vi "Parser Dryer Performance.vi"(8 "error in":errorcluster, 9 "Process Debug?":bool, 10 "log file path in":path=path "C:/faildryer/T00063280_12HL1942_12lb_   COT_R150_ 90IMC_2 - _dlr_run   5_75 50_20120702_1508_DPT.csv", 11 "debug log path in":path=path "C:/test1/dubuglogtest.csv") -> (0 "error out":errorcluster, 2 "new file path out":path)   [LabVIEW 2012]
uses:
  Global Test Variables DPT.vi
  <vilib>/Analysis/baseanly.llb/Mean (DBL).vi
  <vilib>/Utility/file.llb/Write To Spreadsheet File (string).vi
  <vilib>/gmath/NI_Gmath.lvlib
  <vilib>/Analysis/NI_AALBase.lvlib
panel:
  in  "analysis file":path=path "C:/Documents and Settings/JOHN CONWAY/Desktop/Cham 2 Failures/Analysis.csv"
  in  "Write Analysis File":bool
  out "File Name String":string
  out "Compensated - raw":cluster{"Column Data":dbl[], dbl[]}(graph)
  in  "Debug Information":enum32{"Debug Info", "Page 2"}(tab)
  out "Timeing":u32[](array[numeric])
  out "Array":string[](array[string])
  out "Current State":string
  out "Date Time String Array":string[][](array[string])
  out "Debug Time Array":string[](array[string])
  in  "Write Eng File?":bool=TRUE
  in  "Tab Control":T1(tab)=enum."Debug Log"
  out "Data Log File Data In":string[][](array[string])
  out "File Data Out":string[][](array[string])
  in  "Filename Suffix":string="_ENG"
  out "TT4 Extrapolated":bool
  out "RMC Compensated":T2(graph)
  out "Init Moisture Content":dbl
  out "Final Moisture %":dbl
  out "Date String":string
  out "RDB F":T3(graph)
  out "TT 3%":dbl
  out "TT 4%":dbl
  out "TT 5%":dbl
  out "TT3 Extrapolated":bool
  out "TT5 Extrapolated":bool
  out "Gas kWH":T3(graph)
  out "Total kWH":T3(graph)
  out "Heating Val":dbl
  out "Electric kWH":T3(graph)
  out "Total kWH":dbl
  out "Elec kWH":dbl
  out "Gas kWH 2":dbl
  out "Electric Watts":T3(graph)
  out "Gas Watts":T3(graph)
  out "Ave Gas Watts":dbl format="%0.2f"
  out "Ave Elect Watts":dbl format="%0.2f"
  out "Com Count (x(k+1)-x(k))":dbl[](graph)
  out "Debug Data":dbl[][](array[numeric])
  out "Headers for Debug Data":string[](array[string])
  out "error out":errorcluster
  out "Error Indicated in Last 2cols\nof Debug Log":bool
  out "Weight/Raw Weight Data":T2(graph)
  out "FMC (lbs)":dbl
  out "Empty Dryer Wt":dbl
  out "Measured IMC":dbl
  out "FMC %":dbl
  out "FMC (lbs) Predicted":dbl
  out "BDW":dbl
  out "Gas W Data":dynamicdata(graph)
  out "Gas Temp E38":dbl[](array[numeric])
  out "Gas Vol Init E41":dbl
  out "Gas Vol E42":dbl[](array[numeric])
  out "Gas Pres E37":dbl[](array[numeric])
  out "Bar.Pres E36":dbl[](array[numeric])
  out "Header":string[](array[string])
  in  "OK":bool
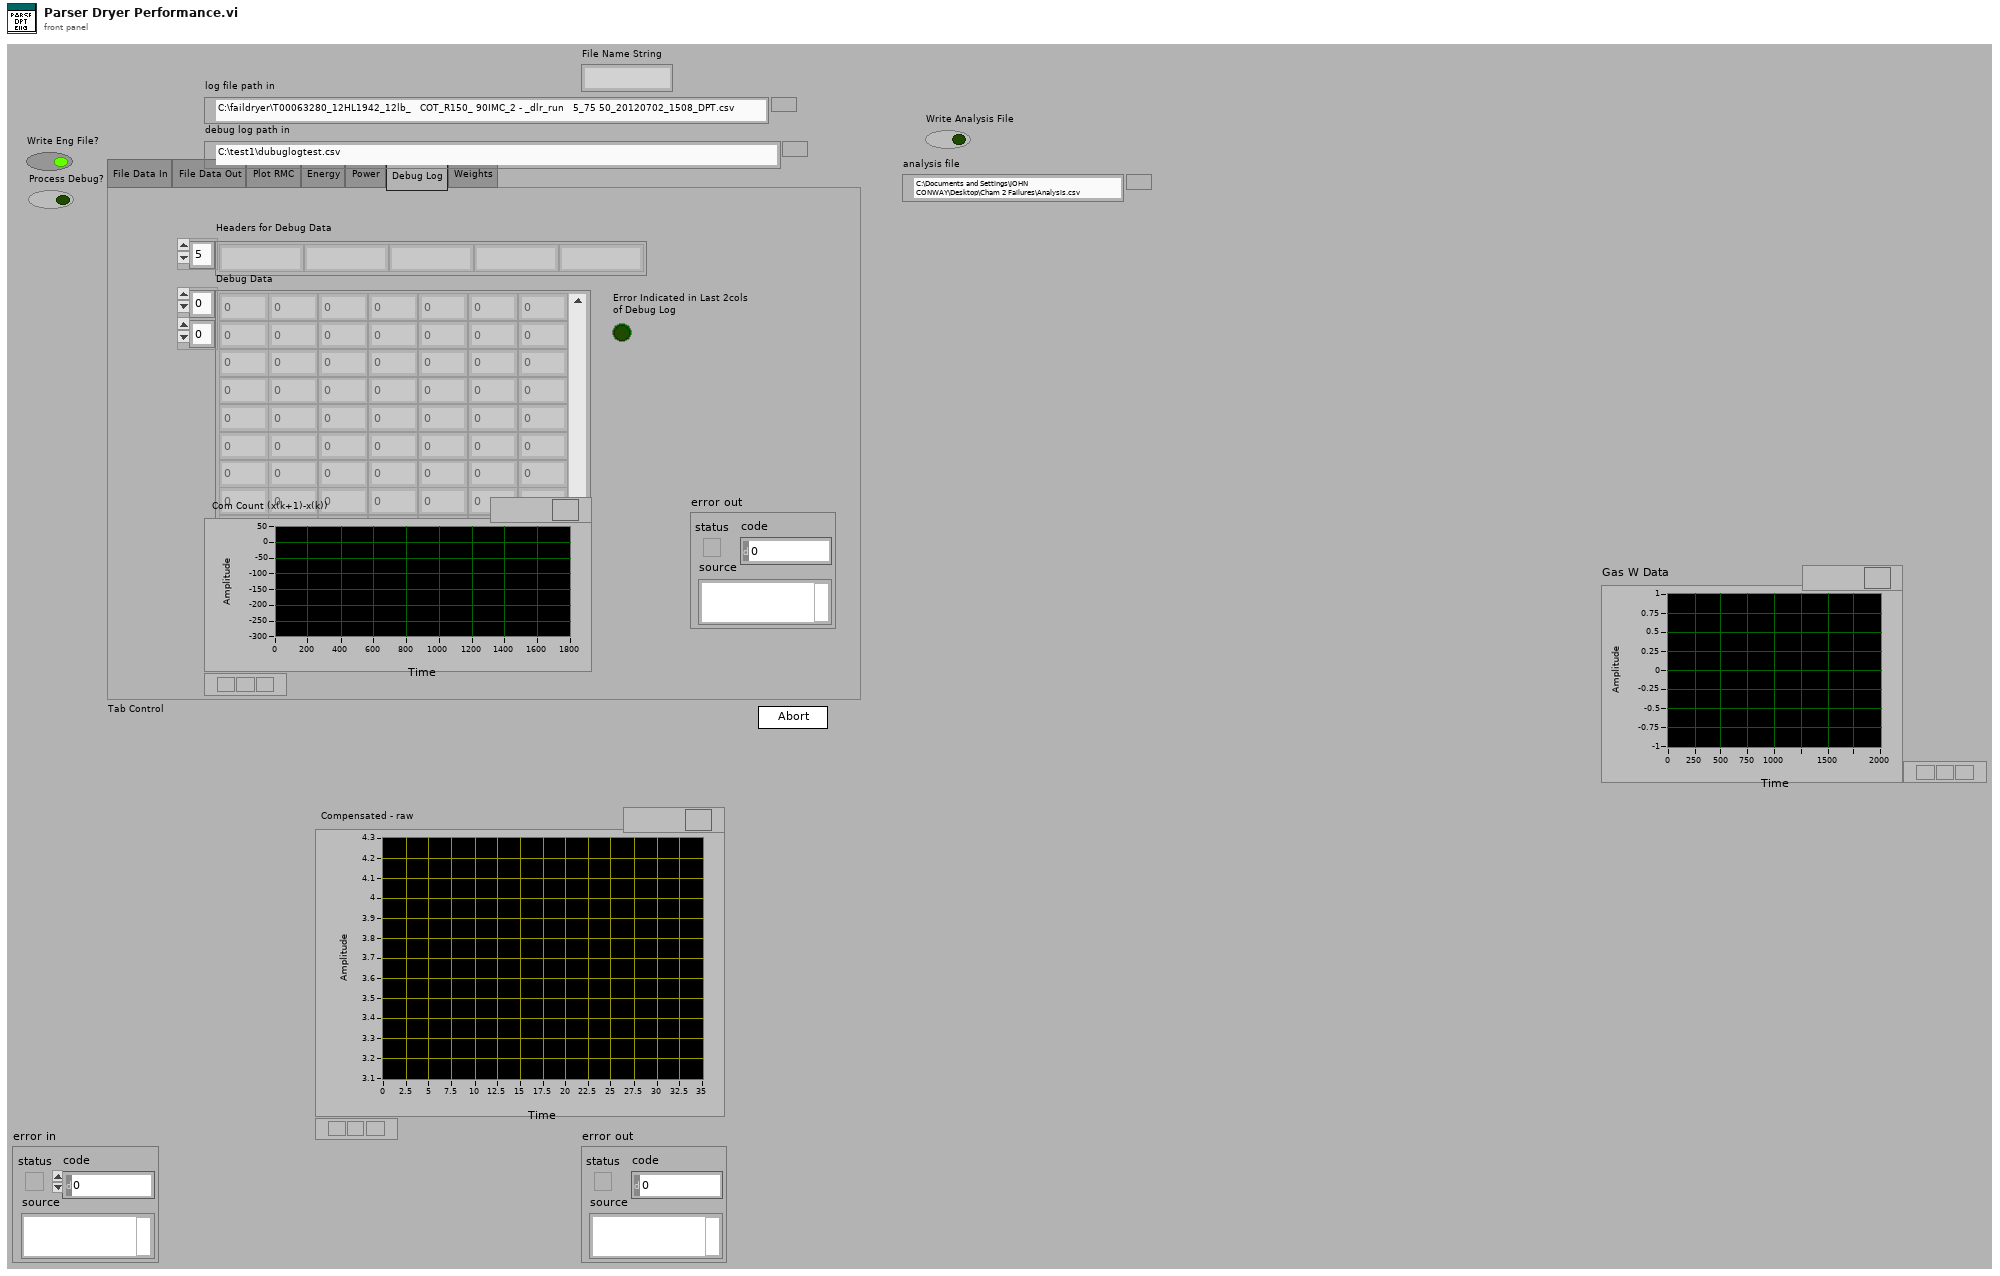
[diagram p1: front panel]
types:
  T1 = enum32{"File Data In", "File Data Out", "Plot RMC", "Energy", "Power", "Debug Log", "Weights"}
  T2 = cluster{"Column Data":dbl[], "Column Data":dbl[]}[]
  T3 = cluster{"Column Data":dbl[], "Column Data":dbl[]}
  T4 = enum32{"invalid app kind", "Development System", "Run Time System", "Student Edition", "Embedded LabVIEW", "Evaluation", "Custom"}
  T5 = enum32{"Invalid", "Standard", "Closed", "Hidden", "Minimized", "Maximized"}
  T6 = cluster{"Core":cluster{"Current VI Reference":refnum<vi>, "Close Panel on Exit?":bool}, "File Data In":string[][], "file path (dialog if empty)":path, "File Data Out":string[][], "Header Labels":string[], "Data":dbl[][], "Logged Data":string[][], "Debug Data In":string[][], "Time Date String Array":string[][], "error in":errorcluster}
  T7 = cluster{"Current VI Reference":refnum<vi>, "Close Panel on Exit?":bool}
  T8 = cluster{"Init Moisture Content":dbl, "Final Moisture %":dbl}
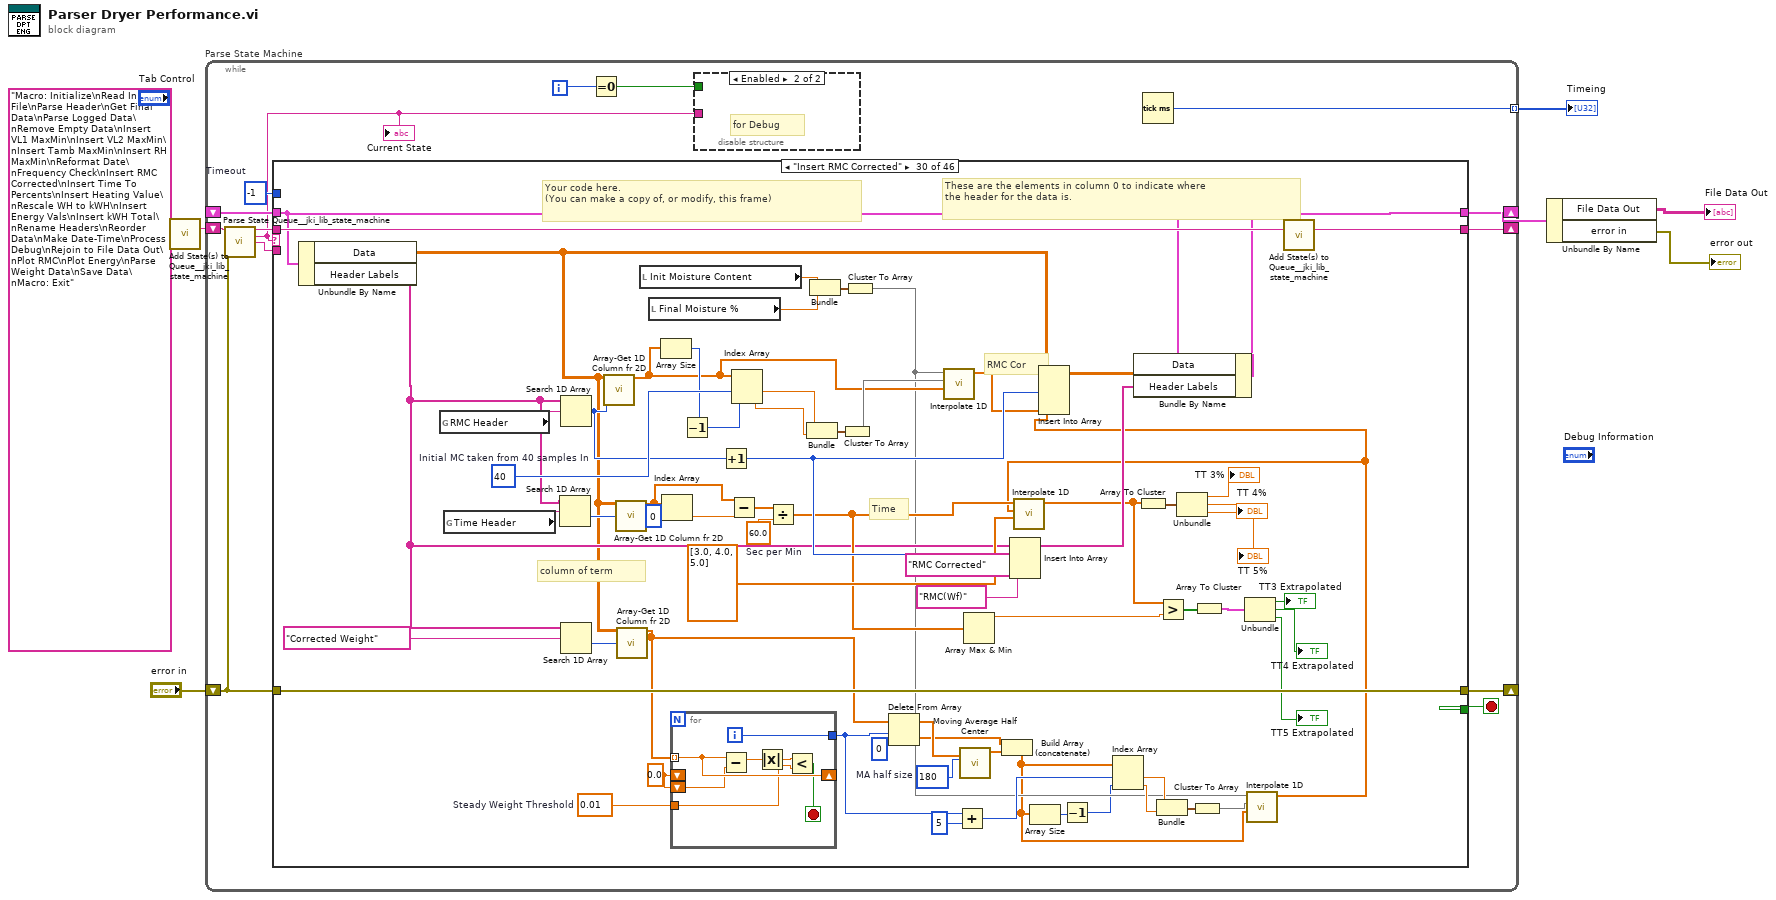
[diagram p0: block diagram]
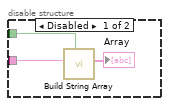
[diagram p2: hidden frame]
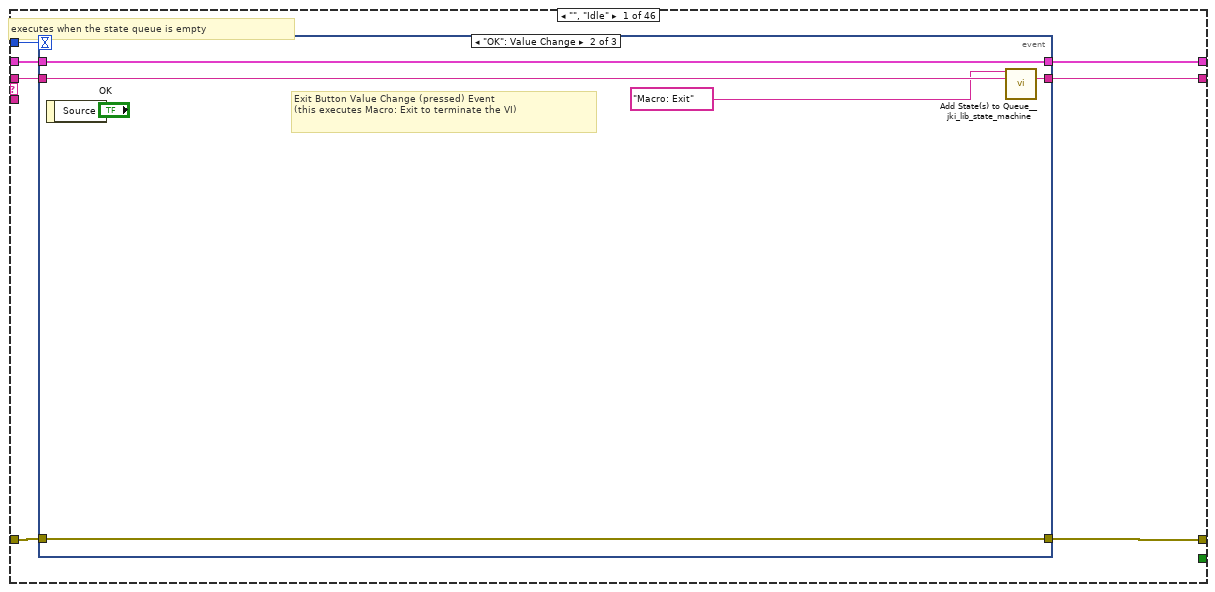
[diagram p3: hidden frame]
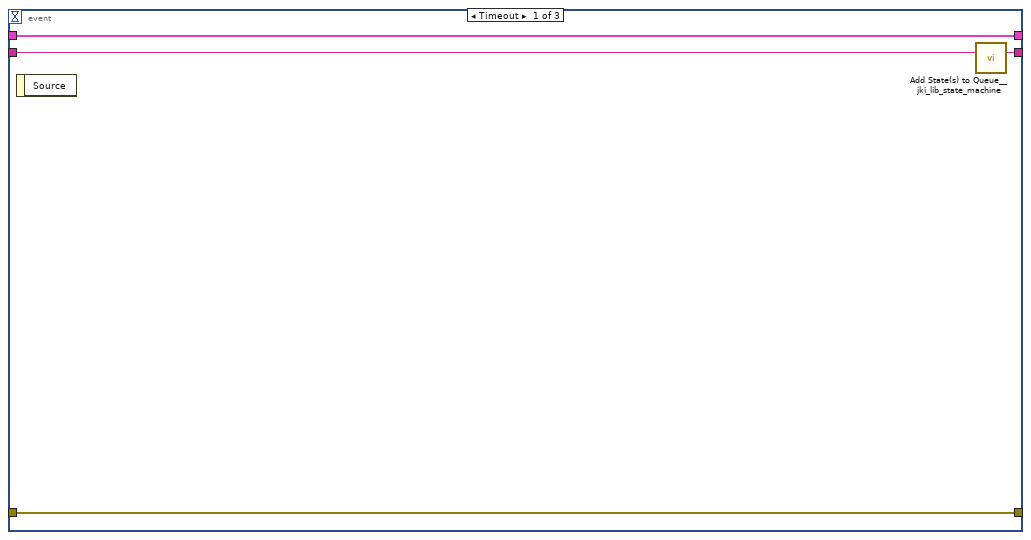
[diagram p4: hidden frame]
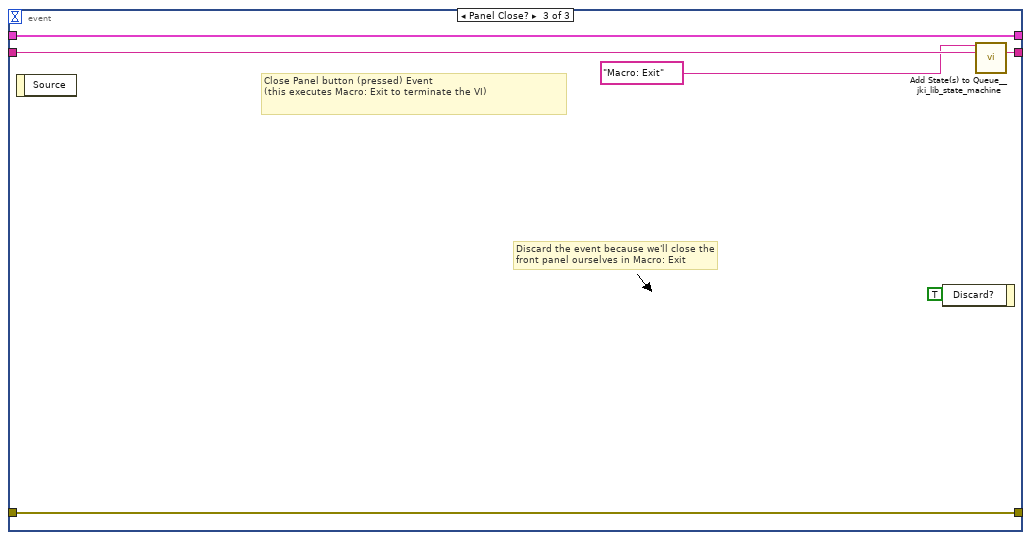
[diagram p5: hidden frame]
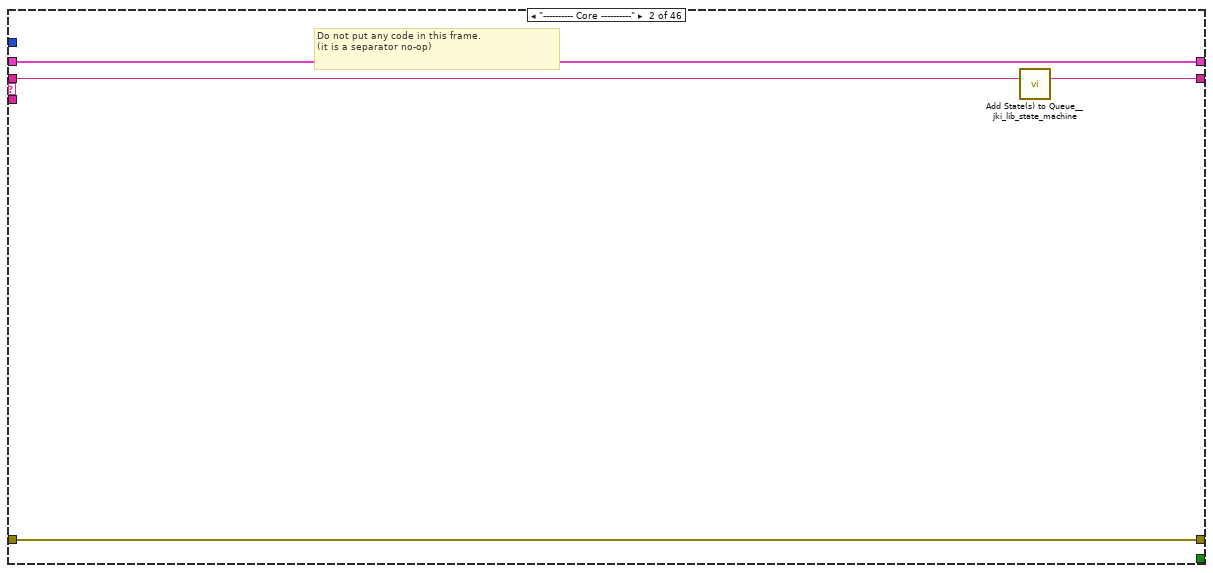
[diagram p6: hidden frame]
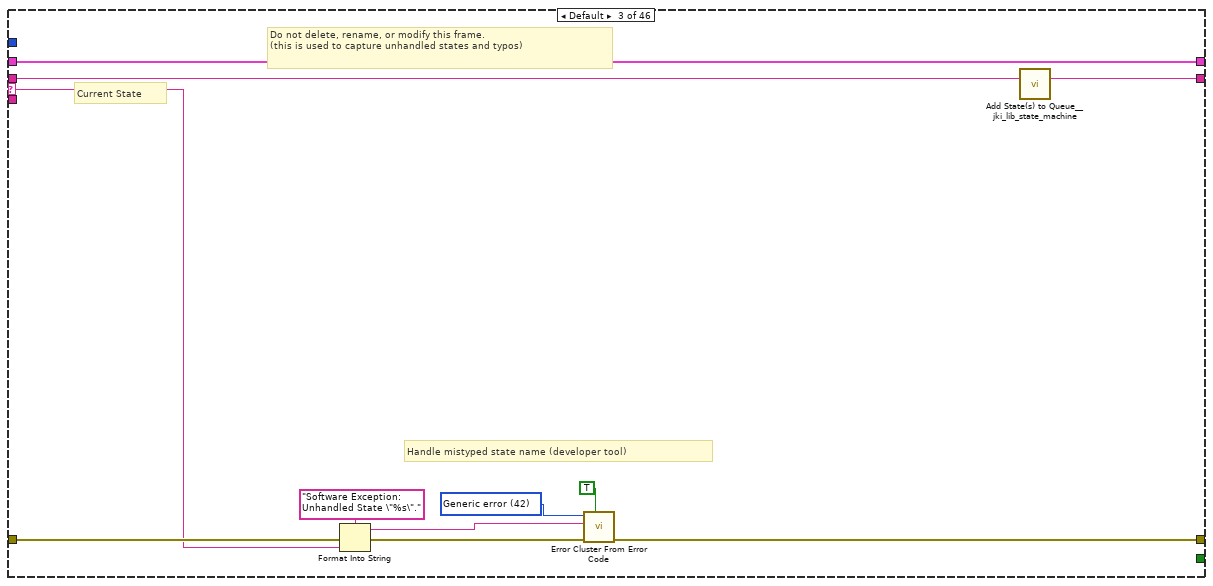
[diagram p7: hidden frame]
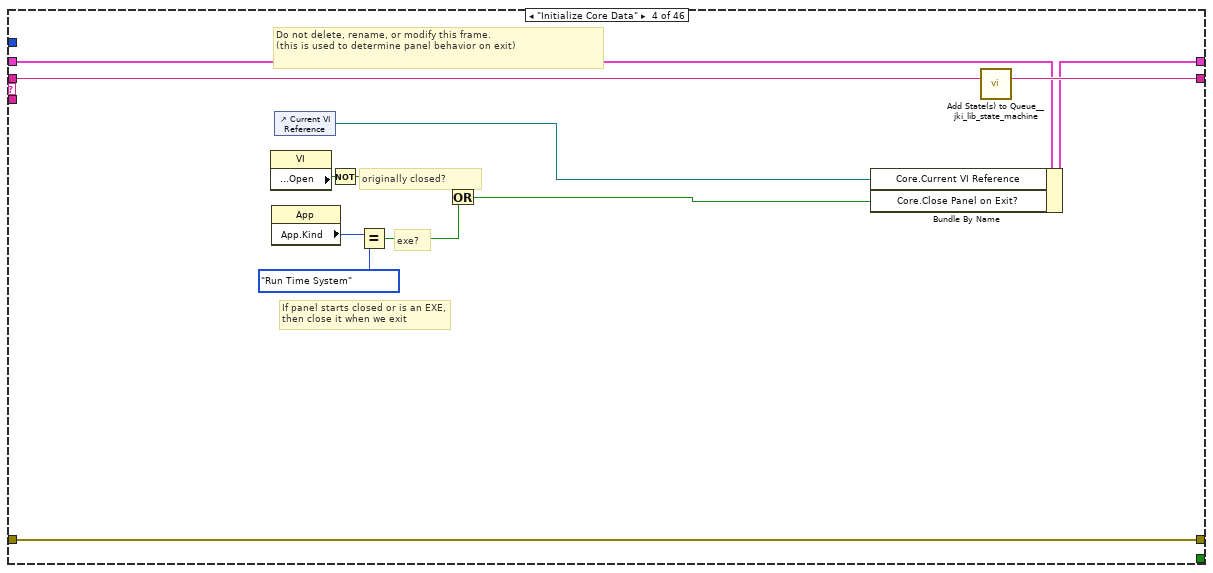
[diagram p8: hidden frame]
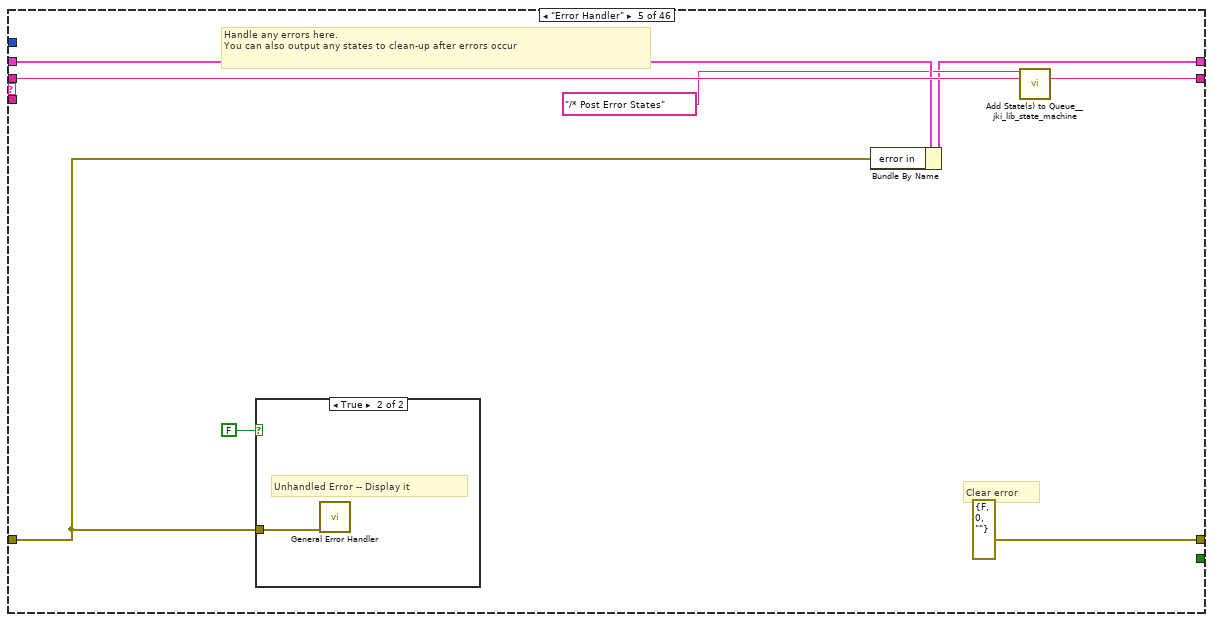
[diagram p9: hidden frame]
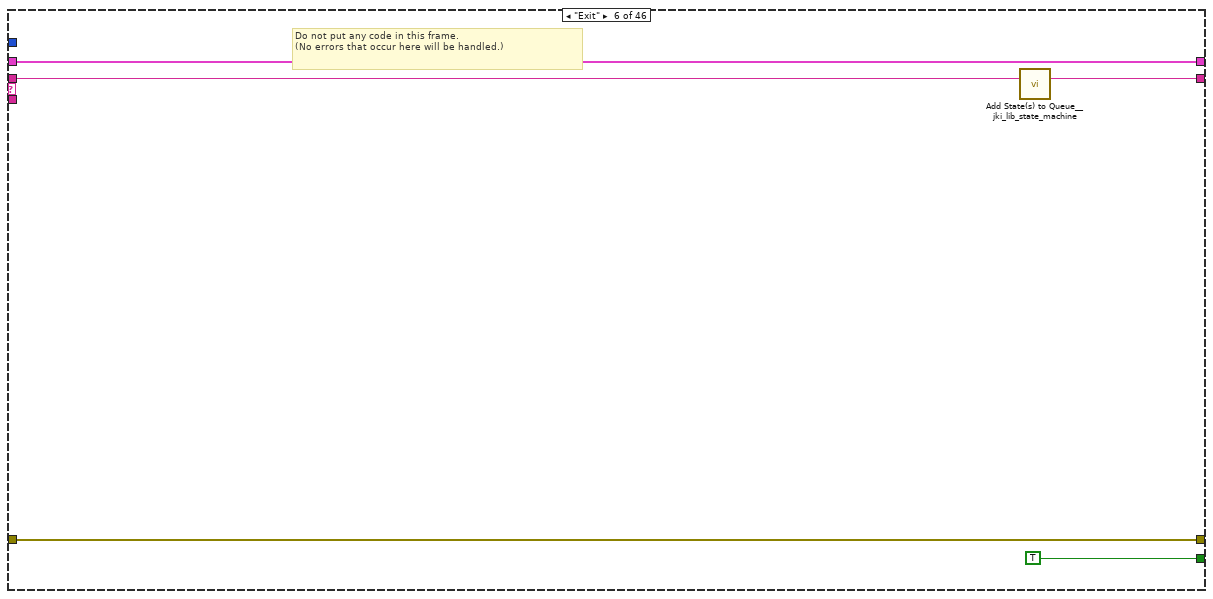
[diagram p11: hidden frame]
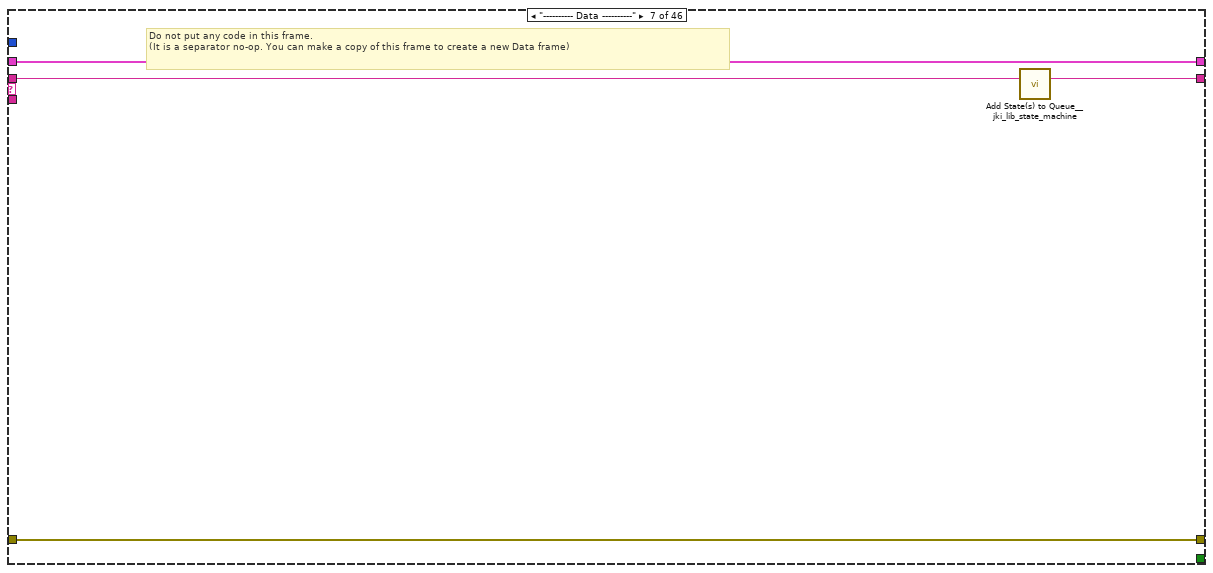
[diagram p12: hidden frame]
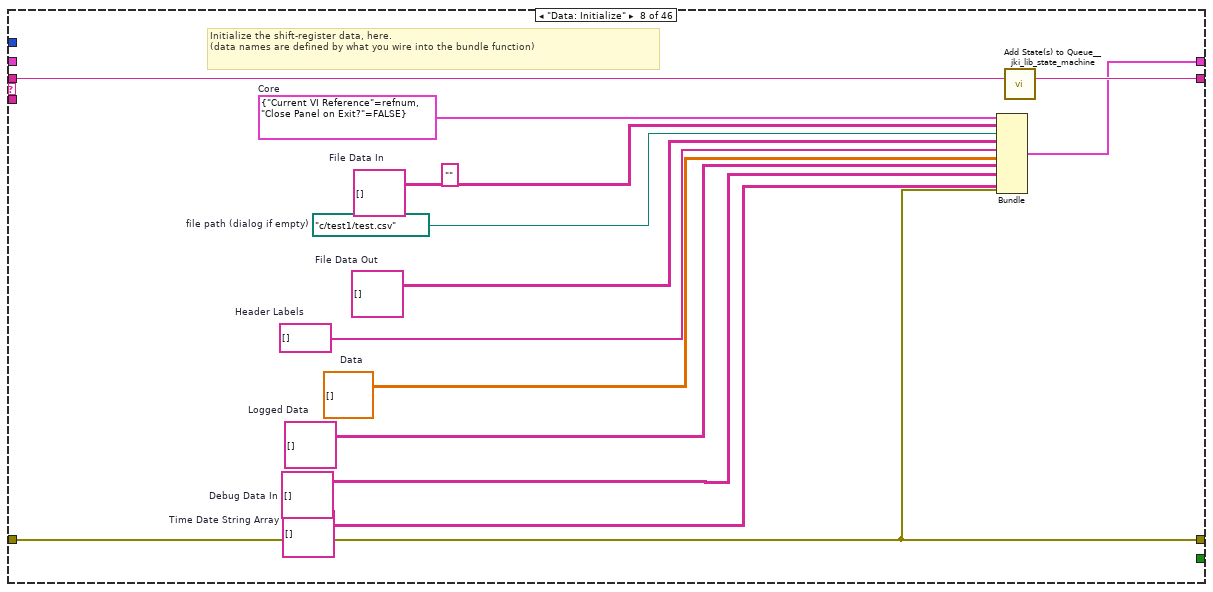
[diagram p13: hidden frame]
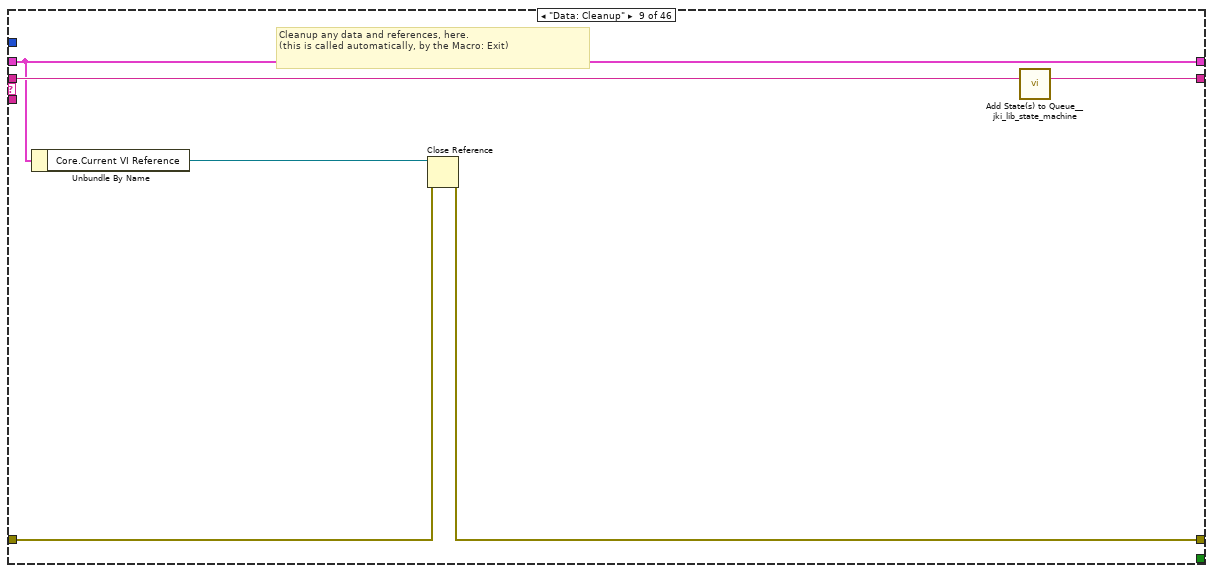
[diagram p14: hidden frame]
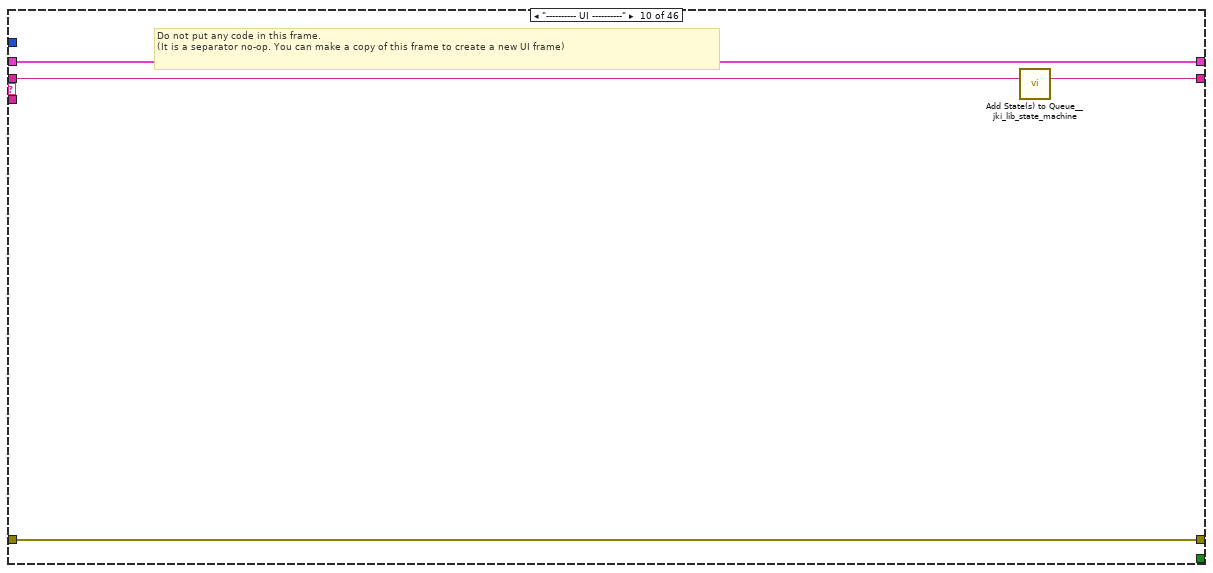
[diagram p15: hidden frame]
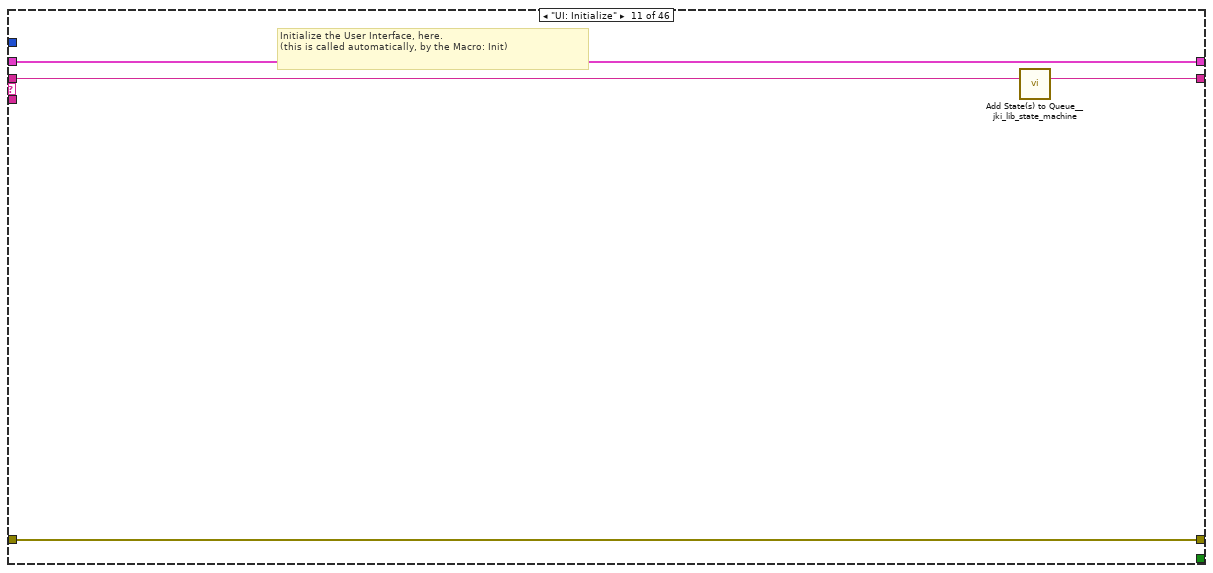
[diagram p16: hidden frame]
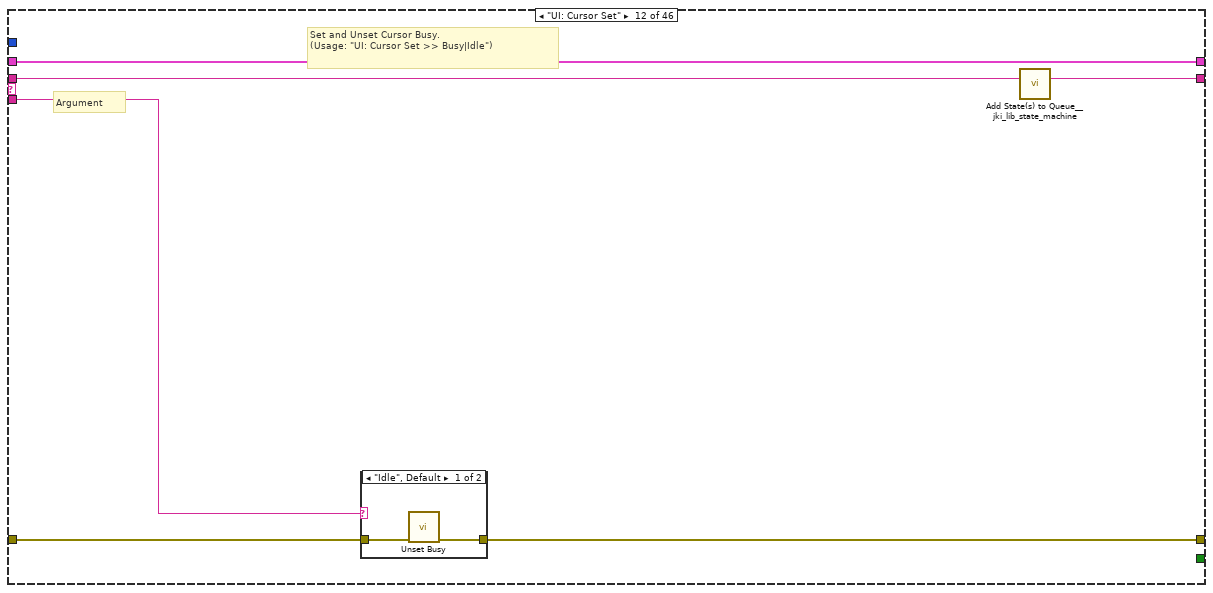
[diagram p17: hidden frame]
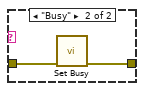
[diagram p18: hidden frame]
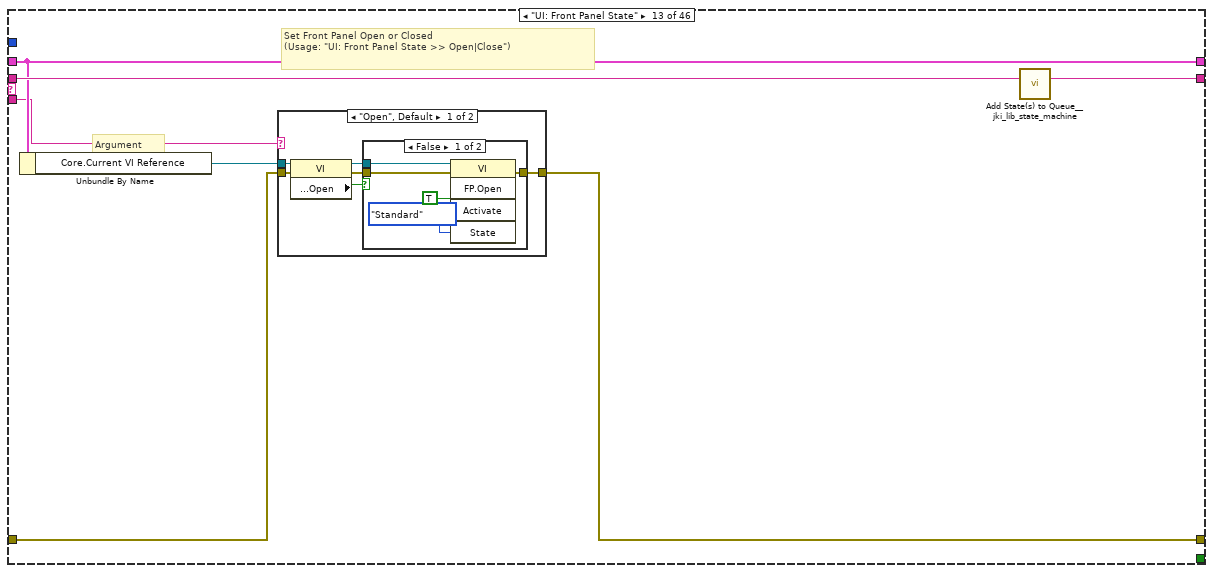
[diagram p19: hidden frame]
diagram:
  n1 = call <vilib>:"Add State(s) to Queue__jki_lib_state_machine.vi"("State(s) in (\"\")"="Macro: Initialize\nRead In Log File\nParse Header\nGet Final Data\nParse Logged Data\nRemove Empty Data\nInsert VL1 MaxMin\nInsert VL2 MaxMin\nInsert Tamb MaxMin\nInsert RH MaxMin\nReformat Date\nFrequency Check\nInsert RMC Corrected\nInsert Time To Percents\nInsert Heating Value\nRescale WH to kWH\nInsert Energy Vals\nInsert kWH Total\nRename Headers\nReorder Data\nMake Date-Time\nProcess Debug\nRejoin to File Data Out\nPlot RMC\nPlot Energy\nParse Weight Data\nSave Data\nMacro: Exit") -> ("States Out"=w7:string)  [unwired: 14 in]
  n2 = while "Parse State Machine" {
    shift-right: [w15] -> w5
    shift-left: _ -> [w14]
    shift-right: [w18] -> _
    shift-left: "error in" -> [w12]
    shift-right: [w17] -> _
    shift-left: w7 -> [w19]
    tunnel: [w8] -> w3 mode=indexing
    i -> [w10]
    stop <- w16 stop-if-true
    w13 = -1  # Timeout
    n3 = call <vilib>:"Parse State Queue__jki_lib_state_machine.vi"("State Queue"=w19, "Error In (no error)"=w12) -> ("Remaining States"=w21:string, "Current State"=w11:string, "Arguments"=w20:string)  [unwired: 11 in]
    "Current State" <- w11
    n4 = case shown="\"Insert RMC Corrected\"" w11 {
      selector: w11 -> [_ _ w51 _ _ _ _ _ _ _ _ _ _ _ _ _ _ _ _ _ _ _ _ _ _ _ _ _ _ _ _ _ _ _ _ _ _ _ _ _ _ _ _ _ _ _]
      tunnel: w21 -> [w31 w50 w55 w73 w81 w87 w91 w104 w110 w114 w118 w124 w135 w161 w166 w176 w180 w190 w207 w264 w285 w400 w433 w475 w501 w527 w553 w575 w590 w664 w700 w716 w729 w785 w803 w811 w832 w915 w932 w960 w994 w1001 w1030 w1036 w1088 w1102]
      tunnel: w20 -> [_ _ _ _ _ _ _ _ _ _ _ w119 w129 _ _ _ _ _ _ _ _ _ _ _ _ _ _ _ _ _ _ _ _ _ _ _ _ _ _ _ _ _ _ _ _ w1092]
      tunnel: w14 -> [w29 w47 w53 w64 w78 w85 w88 _ w105 w111 w116 w122 w131 w158 w163 w173 w177 w187 w194 w257 w282 w365 w425 w457 w483 w509 w535 w556 w581 w648 w697 w709 w723 w781 w799 w808 w829 w912 w929 w957 w991 w998 w1027 w1033 w1085 w1099]
      tunnel: [w28 w48 w57 w70 errorcluster {"status"=FALSE, "code"=0, "source"=""} ("error out") w84 w89 w92 w106 w112 w115 w120 w132 w159 w164 w174 w178 w181 w205 w262 w283 w398 w431 w473 w499 w525 w551 w573 w588 w662 w698 w714 w727 w783 w801 w809 w830 w913 w930 w958 w992 w999 w1028 w1034 w1086 w1100] -> w18
      tunnel: w12 -> [w27 w48 w56 w70 w75 w84 w89 w92 w107 w112 w115 w121 w133 w159 w164 w174 w178 w182 w205 w262 w283 w398 w431 w473 w499 w525 w551 w573 w588 w662 w698 w714 w727 w783 w801 w809 w830 w913 w930 w958 w992 w999 w1028 w1034 w1086 w1100]
      tunnel: [w30 w49 w54 w72 w80 w86 w90 w103 w109 w113 w117 w123 w134 w160 w165 w175 w179 w189 w206 w263 w284 w399 w432 w474 w500 w526 w552 w574 w589 w663 w699 w715 w728 w784 w802 w810 w831 w914 w931 w959 w993 w1000 w1029 w1035 w1087 w1101] -> w17
      tunnel: [_ _ _ _ _ TRUE _ _ _ _ _ _ _ _ _ _ _ _ _ _ _ _ _ _ _ _ _ _ _ _ _ _ _ _ _ _ _ _ _ _ _ _ _ _ _ _] -> w16
      tunnel: [w26 w47 w53 w71 w76 w85 w88 w102 w105 w111 w116 w122 w131 w158 w163 w173 w177 w186 w193 w256 w281 w365 w424 w457 w483 w509 w535 w557 w582 w647 w697 w708 w722 w780 w798 w807 w828 w911 w928 w957 w991 w998 w1027 w1032 w1085 w1098] -> w15
      tunnel: w13 -> [w25 _ _ _ _ _ _ _ _ _ _ _ _ _ _ _ _ _ _ _ _ _ _ _ _ _ _ _ _ _ _ _ _ _ _ _ _ _ _ _ _ _ _ _ _ _]
      frame "", "Idle" {
        # "executes when the state queue is empty"
        n5 = event shown="[1] \"OK\": Value Change" {
          selector: _ -> [_ _ _]
          dyn-events: _ -> [_ _ _]
          timeout: w25 -> [_ _ _]
          tunnel: w31 -> [w35 w40 w46]
          tunnel: [w34 w39 w45] -> w30
          tunnel: w29 -> [w32 w37 w43]
          tunnel: [w33 w38 w44] -> w28
          tunnel: w27 -> [w33 w38 w44]
          tunnel: [w32 w37 w43] -> w26
          event Timeout {
            n6 = event-data() -> ()  [unwired: 1 in, 1 out]
            n7 = call <vilib>:"Add State(s) to Queue__jki_lib_state_machine.vi"("State(s) in (\"\")"=w35) -> ("States Out"=w34:string)  [unwired: 14 in]
          }
          event "OK": Value Change {
            # "Exit Button Value Change (pressed) Event\n(this executes Macro: Exit to terminate the VI)"
            n8 = event-data() -> ()  [unwired: 1 in, 1 out]
            n9 = call <vilib>:"Add State(s) to Queue__jki_lib_state_machine.vi"("State(s) in Front (\"\")"="Macro: Exit", "State(s) in (\"\")"=w40) -> ("States Out"=w39:string)  [unwired: 13 in]
          }
          event Panel Close? {
            # "Discard the event because we'll close the front panel ourselves in Macro: Exit"
            # "Close Panel button (pressed) Event\n(this executes Macro: Exit to terminate the VI)"
            n10 = event-data() -> ()  [unwired: 1 in, 1 out]
            n11 = event-data("Discard?"=TRUE) -> ()  [unwired: 1 in, 1 out]
            n12 = call <vilib>:"Add State(s) to Queue__jki_lib_state_machine.vi"("State(s) in Front (\"\")"="Macro: Exit", "State(s) in (\"\")"=w46) -> ("States Out"=w45:string)  [unwired: 13 in]
          }
        }
      }
      frame "---------- Core ----------" {
        # "Do not put any code in this frame.\n(it is a separator no-op)"
        n13 = call <vilib>:"Add State(s) to Queue__jki_lib_state_machine.vi"("State(s) in (\"\")"=w50) -> ("States Out"=w49:string)  [unwired: 14 in]
      }
      frame Default {
        w60 = 42 items=["No error", "Argument error", "Memory is full", "Out of zone", "End of file", "File already open", "Generic file I/O error", "File not found", "File permission error", "Disk is full", "Duplicate path", "Too many files open", "System feature not enabled", "Resource file not found", "Cannot add resource", "Resource not found", "Image not found", "Image memory error", "Pen does not exist", "Config type invalid", "Config token not found", "Config parse error", "Config memory error", "Bad external code format", "Bad external code offset", "External code not present", "Null window", "Destroy window error", "Null menu", "Print aborted", "Bad print record", "Print driver error", "Windows error during printing", "Memory error during printing", "Print dialog error", "Generic print error", "Invalid device refnum", "Device not found", "Device parameter error", "Device unit error", "Cannot open device", "Device call aborted", "Generic error", "Cancelled by user", "Object ID too low", "Object ID too high", "Object not in heap", "Unknown heap", "Unknown object (invalid DefProc)", "Unknown object (DefProc not in table)", "Message out of range", "Invalid (null) method", "Unknown message", "Manager call not supported", "Bad address", "Network operation in progress", "Network operation timed out", "Connection is busy", "Network attribute not supported", "Network error", "Address in use", "System out of memory", "Connection aborted", "Connection refused", "Not connected", "Already connected", "Connection closed", "Initialization error (interapplication manager)", "Bad occurrence", "Wait on unbound occurrence handler", "Occurrence queue overflow", "Datalog type conflict", "Unused", "Unrecognized type (interapplication manager)", "Memory corrupt", "Failed to make temporary DLL", "Old CIN version", "Drag socket not found", "Failed to load drop-object", "Failed to register OLE object", "Failed to release OLE object", "Format specifier type mismatch", "Unknown format specifier", "Too few format specifiers", "Too many format specifiers", "Scan failed", "Newer CIN version", "Error converting to variant", "Runtime menu error", "Password tampered", "Variant attribute not found", "Incompatible variant data type", "Event data is not available", "Event Store is not present", "Occurrence is not found", "Event Queue is not created", "Event info is not available", "Refnum passed is NULL", "Error retrieving Class GUID", "Error retrieving CoClass GUID", "Error retrieving TypeLib GUID.", "Bad built application magic bytes.", "Specific driver is different from the specific driver associated with the Logical Name.", "There is no session opened to the class driver.", "Max Error", "MAX - Error with config objects", "MAX - Error loading configuration", "MAX - Group not supported"]
        # "Current State"
        # "Do not delete, rename, or modify this frame.\n(this is used to capture unhandled states and typos)"
        # "Handle mistyped state name (developer tool)"
        n14 = Format Into String(format string="Software Exception: Unhandled State \"%s\"." ("message"), error in=w56, w51) -> (resulting string=w59:string, error out=w58:errorcluster)  [unwired: 1 in]
        n15 = call <vilib>:"Error Cluster From Error Code.vi"("show call chain? (False)"=TRUE, "error in (no error)"=w58, "error message (\"\")"=w59, "error code (0)"=w60) -> ("error out"=w57:errorcluster)  [unwired: 5 in]
        n16 = call <vilib>:"Add State(s) to Queue__jki_lib_state_machine.vi"("State(s) in (\"\")"=w55) -> ("States Out"=w54:string)  [unwired: 14 in]
      }
      frame "Initialize Core Data" {
        # "Do not delete, rename, or modify this frame.\n(this is used to determine panel behavior on exit)"
        # "originally closed?"
        # "exe?"
        # "If panel starts closed or is an EXE, then close it when we exit"
        n17 = property class="VI"() -> ("Front Panel.Open"=w69:bool)  [unwired: 2 in, 2 out]
        n18 = property class="App"() -> ("App.Kind"=w68:T4)  [unwired: 2 in, 2 out]
        n19 = control-ref of="Current VI Reference"() -> (w62:refnum<vi>)
        n20 = Not(x=w69) -> (.not. x?=w66:bool)
        n21 = Equal?(x=w68, y=T4."Run Time System" ("Application:Kind")) -> (x = y?=w65:bool)
        n22 = Or(x=w66, y=w65) -> (x .or. y?=w63:bool)
        n23 = Bundle By Name(cluster=w64, "Core.Current VI Reference"=w62, "Core.Close Panel on Exit?"=w63) -> (w71:T6)
        n24 = call <vilib>:"Add State(s) to Queue__jki_lib_state_machine.vi"("State(s) in (\"\")"=w73) -> ("States Out"=w72:string)  [unwired: 14 in]
      }
      frame "Error Handler" {
        # "Handle any errors here.\nYou can also output any states to clean-up after errors occur"
        # "Clear error"
        n25 = case shown="True" FALSE {
          tunnel: w75 -> [_ w82]
          frame False {
          }
          frame True {
            # "Unhandled Error -- Display it"
            n26 = call <vilib>:"General Error Handler.vi"("error in (no error)"=w82) -> ()  [unwired: 10 in, 5 out]
          }
        }
        n27 = Bundle By Name(cluster=w78, "error in"=w75) -> (w76:T6)
        n28 = call <vilib>:"Add State(s) to Queue__jki_lib_state_machine.vi"("State(s) in Front (\"\")"="/* Post Error States", "State(s) in (\"\")"=w81) -> ("States Out"=w80:string)  [unwired: 13 in]
      }
      frame "Exit" {
        # "Do not put any code in this frame.\n(No errors that occur here will be handled.)"
        n29 = call <vilib>:"Add State(s) to Queue__jki_lib_state_machine.vi"("State(s) in (\"\")"=w87) -> ("States Out"=w86:string)  [unwired: 14 in]
      }
      frame "---------- Data ----------" {
        # "Do not put any code in this frame.\n(It is a separator no-op. You can make a copy of this frame to create a new Data frame)"
        n30 = call <vilib>:"Add State(s) to Queue__jki_lib_state_machine.vi"("State(s) in (\"\")"=w91) -> ("States Out"=w90:string)  [unwired: 14 in]
      }
      frame "Data: Initialize" {
        w93 = string[][] []  # Time Date String Array
        w94 = string[][] []  # Debug Data In
        w95 = string[][] []  # Logged Data
        (unwired) "" ("String")
        w96 = dbl[][] []  # Data
        w97 = string[] []  # Header Labels
        w98 = string[][] []  # File Data Out
        w99 = path "c:/test1/test.csv"  # file path (dialog if empty)
        w100 = string[][] []  # File Data In
        w101 = T7 {"Current VI Reference"=refnum, "Close Panel on Exit?"=FALSE}  # Core
        # "Initialize the shift-register data, here.\n(data names are defined by what you wire into the bundle function)"
        n31 = Bundle("Core"=w101, "File Data In"=w100, "file path (dialog if empty)"=w99, "File Data Out"=w98, "Header Labels"=w97, "Data"=w96, "Logged Data"=w95, "Debug Data In"=w94, "Time Date String Array"=w93, "error in"=w92) -> (w102:T6)  [unwired: 1 in]
        n32 = call <vilib>:"Add State(s) to Queue__jki_lib_state_machine.vi"("State(s) in (\"\")"=w104) -> ("States Out"=w103:string)  [unwired: 14 in]
      }
      frame "Data: Cleanup" {
        # "Cleanup any data and references, here.\n(this is called automatically, by the Macro: Exit)"
        n33 = Unbundle By Name(w105) -> ("Core.Current VI Reference"=w108:refnum<vi>)
        n34 = Close Reference(reference=w108, error in (no error)=w107) -> (error out=w106:errorcluster)
        n35 = call <vilib>:"Add State(s) to Queue__jki_lib_state_machine.vi"("State(s) in (\"\")"=w110) -> ("States Out"=w109:string)  [unwired: 14 in]
      }
      frame "---------- UI ----------" {
        # "Do not put any code in this frame.\n(It is a separator no-op. You can make a copy of this frame to create a new UI frame)"
        n36 = call <vilib>:"Add State(s) to Queue__jki_lib_state_machine.vi"("State(s) in (\"\")"=w114) -> ("States Out"=w113:string)  [unwired: 14 in]
      }
      frame "UI: Initialize" {
        # "Initialize the User Interface, here.\n(this is called automatically, by the Macro: Init)"
        n37 = call <vilib>:"Add State(s) to Queue__jki_lib_state_machine.vi"("State(s) in (\"\")"=w118) -> ("States Out"=w117:string)  [unwired: 14 in]
      }
      frame "UI: Cursor Set" {
        # "Argument"
        # "Set and Unset Cursor Busy.\n(Usage: \"UI: Cursor Set >> Busy|Idle\")"
        n38 = case shown="\"Idle\", Default" w119 {
          tunnel: w121 -> [w126 w128]
          tunnel: [w125 w127] -> w120
          frame "Idle", Default {
            n39 = call <vilib>:"Unset Busy.vi"("error in (no error)"=w126) -> ("error out"=w125:errorcluster)  [unwired: 10 in]
          }
          frame "Busy" {
            n40 = call <vilib>:"Set Busy.vi"("error in (no error)"=w128) -> ("error out"=w127:errorcluster)  [unwired: 9 in, 1 out]
          }
        }
        n41 = call <vilib>:"Add State(s) to Queue__jki_lib_state_machine.vi"("State(s) in (\"\")"=w124) -> ("States Out"=w123:string)  [unwired: 14 in]
      }
      frame "UI: Front Panel State" {
        # "Argument"
        # "Set Front Panel Open or Closed\n(Usage: \"UI: Front Panel State >> Open|Close\")"
        n42 = Unbundle By Name(w131) -> ("Core.Current VI Reference"=w130:refnum<vi>)
        n43 = case shown="\"Open\", Default" w129 {
          tunnel: w133 -> [w139 w152]
          tunnel: [w141 w153] -> w132
          tunnel: w130 -> [w140 w150]
          frame "Open", Default {
            n44 = property class="VI"(reference=w140, error in=w139) -> (reference out=w137:refnum<vi>, error out=w138:errorcluster, "Front Panel.Open"=w136:bool)
            n45 = case shown="False" w136 {
              tunnel: [w144 w147] -> w141
              tunnel: w138 -> [w143 w147]
              tunnel: w137 -> [w142 _]
              frame False {
                n46 = invoke class="VI" method="FP.Open"(reference=w142, error in=w143, "Activate"=TRUE, "State"=T5."Standard") -> (error out=w144:errorcluster)  [unwired: 1 in, 4 out]
              }
              frame True {
              }
            }
          }
          frame "Close" {
            n47 = property class="VI"(reference=w150, error in=w152) -> (reference out=w149:refnum<vi>, error out=w151:errorcluster, "Front Panel.Open"=w148:bool)
            n48 = case shown="True" w148 {
              tunnel: [w154 w157] -> w153
              tunnel: w151 -> [w154 w156]
              tunnel: w149 -> [_ w155]
              frame False {
              }
              frame True {
                n49 = invoke class="VI" method="FP.Close"(reference=w155, error in=w156) -> (error out=w157:errorcluster)  [unwired: 1 in, 2 out]
              }
            }
          }
        }
        n50 = call <vilib>:"Add State(s) to Queue__jki_lib_state_machine.vi"("State(s) in (\"\")"=w135) -> ("States Out"=w134:string)  [unwired: 14 in]
      }
      frame "---------- Macro ----------" {
        # "Do not put any code in this frame.\n(It is a separator no-op. You can make a copy of this frame to create a new Macro frame)"
        n51 = call <vilib>:"Add State(s) to Queue__jki_lib_state_machine.vi"("State(s) in (\"\")"=w161) -> ("States Out"=w160:string)  [unwired: 14 in]
      }
      frame "Macro: Initialize" {
        # "Initialization Macro\n(This is called once, when the VI starts)"
        n52 = call <vilib>:"Add State(s) to Queue__jki_lib_state_machine.vi"("State(s) in Front (\"\")"="Data: Initialize\nInitialize Core Data\nUI: Initialize", "State(s) in (\"\")"=w166) -> ("States Out"=w165:string)  [unwired: 13 in]
      }
      frame "Macro: Exit" {
        # "Exit Macro\n(This is called once, when the VI exits)"
        n53 = Unbundle By Name(w173) -> ("Core.Close Panel on Exit?"=w172:bool)
        n54 = Select(t="UI: Front Panel State >> Close", s=w172, f="") -> (s? t:f=w169:string)
        n55 = call <vilib>:"Add State(s) to Queue__jki_lib_state_machine.vi"("State(s) in (\"\")"=w169, "State(s) at Back (\"\")"="Data: Cleanup\nExit") -> ("States Out"=w167:string)  [unwired: 13 in]
        n56 = call <vilib>:"Add State(s) to Queue__jki_lib_state_machine.vi"("State(s) in Front (\"\")"=w167, "State(s) in (\"\")"=w176) -> ("States Out"=w175:string)  [unwired: 13 in]
      }
      frame "---------- Main ----------" {
        # "Template Separator\n(You can make a copy of, or modify, this frame)"
        n57 = call <vilib>:"Add State(s) to Queue__jki_lib_state_machine.vi"("State(s) in (\"\")"=w180) -> ("States Out"=w179:string)  [unwired: 14 in]
      }
      frame "Read In Log File" {
        n58 = Strip Path(path="log file path in") -> (name=→"File Name String":string)  [unwired: 1 out]
        n59 = call "Read From Spreadsheet File (string) with Error.vi"("delimiter (\\t)"="," ("delimiter (\\t)"), "error in"=w182, "file path (dialog if empty)"="log file path in") -> ("error out"=w181:errorcluster, "all rows"=w185:string[][])  [unwired: 4 in, 3 out]
        "Data Log File Data In" <- w185
        n60 = Bundle By Name(cluster=w187, "File Data In"=w185) -> (w186:T6)
        n61 = call <vilib>:"Add State(s) to Queue__jki_lib_state_machine.vi"("State(s) in (\"\")"=w190) -> ("States Out"=w189:string)  [unwired: 14 in]
      }
      frame "Parse Header" {
        w195 = "TEST STATION:\t&Station \nCOMPUTER_NAME:\t&Computername\nVERSION:\t&Version\nTR_NUMBER:\t&TR#\nENGINEER:\t&Engineer\nTECHNICIAN:\t&Tech\nFILENAME:\t&Filename\nCOMMENTS:\t&Comments\nDATE:\t&Date\nBuild\t&Build\nLAB ID:\t&Unit\nMODEL:\t&Model\nSerial Number\t&Serial\nDRYER TYPE\t&Dryer Type\nSUPPLY VOLTAGE:\t&Voltage\nFrequency:\t&Freq\nDrum Volume\t&Volume\nTEST_TYPE:\t&Test Type\nTEST_TITLE:\t&Title\nTEST NUM:\t&Test Number\nNom Load Type\t&Load Type\nNom Load Weight\t&Load Size\nLOAD RUN NUM:\t&Run\nDRYING CYCLE:\t&Drying Cycle\nHeat Setting\t&Heat Setting\nDryness Setting\t&Dryness setting\nEXHAUST:\t&Restriction\nBone Dry Wt\t&BDW\nFMC DELAY (min):\t&FMCDelay\nAMBIENT TEMP:\t&AmbTemp\nAMBIENT RH:\t&RH\nRMC Actual\t&IMC\nMeasured IMC\t&InitialWeight\nHeating Val. (BTU/ft3)\t&HeatVal\nEmpty Dryer Cold Weight\t&MTDryer"  # Label, replace string
        w204 = "" ("format string")
        w196 = "" ("format string")
        w201 = "STATION / NAME:\t&Station / &Computername\nVERSION:\t&Version\n--------------------------\t--------------------------\nTR #:\t&TR#\nENGINEER:\t&Engineer\nTECHNICIAN:\t&Tech\n--------------------------\t--------------------------\nFILENAME:\t&Filename\nCOMMENTS:\t&Comments\nDATE:\t&Date\n--------------------------\t--------------------------\nBUILD:\t&Build\nUNIT:\t&Unit\nMODEL #:\t&Model\nSERIAL #:\t&Serial\nDRYER TYPE:\t&Dryer Type\nSUPPLY VOLTAGE:\t&Voltage\nFREQUENCY (Hz):\t&Freq\nDRUM VOL (cuft):\t&Volume\n--------------------------\t--------------------------\nTEST TYPE:\t&Test Type\nTEST TITLE:\t&Title\nTEST #:\t&Test Number\nLOAD TYPE:\t&Load Type\nLOAD SIZE (lbs):\t&Load Size\nLOAD RUN #:\t&Run\n--------------------------\t--------------------------\nDRYING CYCLE:\t&Drying Cycle\nHEAT SETTING:\t&Heat Setting\nDRYNESS SETTING:\t&Dryness setting\nRESTRICTION:\t&Restriction\nBONE DRY WT (lbs):\t&BDW\nINITIAL WT (lbs):\t&InitialWeight\nFINAL WT (lbs):\t&FinalWeight\nIMC:\t&IMC\nFMC:\t&FMC\nFMC DELAY (min):\t&FMCDelay\n--------------------------\t--------------------------\nAMB TEMP (F):\t&AmbTemp\nAMB RH (%):\t&RH\nAMB TEMP (Max / Min):\t&TempMaxMin\nAMB RH (Max / Min):\t&RHMaxMin\nVOLTAGE L1 (Max / Min):\t&VL1MaxMin\nVOLTAGE L2 (Max / Min):\t&VL2MaxMin\n--------------------------\t--------------------------\nTIME TO 5% RMC:\t&TT5\nTIME TO 4% RMC:\t&TT4\nTIME TO 3% RMC:\t&TT3\n--------------------------\t--------------------------"  # ProtoData
        # "Use this loop\nto parse out data used in calculations later."
        # "File Data Out will hold the header info..."
        # "Your code here.\nKeep BDW for use in later calc"
        n62 = Unbundle By Name(w194) -> ("File Data In"=w192:string[][])
        n63 = Delete From Array(array=w192, index (col)=0 ("disabled index (col)")) -> (deleted portion=w198:string[])  [unwired: 2 in, 1 out]
        n64 = Delete From Array(array=w192, index (col)=1 ("disabled index (col)")) -> (deleted portion=w200:string[])  [unwired: 2 in, 1 out]
        n65 = Spreadsheet String To Array(format string=w196, spreadsheet string=w195, array type (2D Dbl)=w196) -> (array=w202:string[][])  [unwired: 1 in]
        n66 = for {
          tunnel: w198 -> [w218]
          tunnel: w200 -> [w216]
          tunnel: w202 -> [w214] mode=indexing
          shift-right: [w210] -> w203
          shift-left: w201 -> [w215]
          # "search header"
          # "replace string"
          n67 = Index Array(array=w214, index #1=0 ("index"), index #2=1 ("index")) -> (element #1=w211:string, element #2=w209:string)
          n68 = Search 1D Array(1D array=w218, element=w211) -> (index of element=w217:i32)  [unwired: 1 in]
          n69 = Index Array(array=w216, index=w217) -> (element=w208:string)
          n70 = case shown="\"False\", Default" w209 {
            tunnel: w208 -> [_ w220 w222 w224 w226 w228]
            frame "False", Default {
            }
            frame "&BDW" {
              n71 = Fract/Exp String To Number(string=w220) -> (number=→"BDW":dbl)  [unwired: 3 in, 1 out]
            }
            frame "&IMC" {
              n72 = Fract/Exp String To Number(string=w222) -> (number=→"Init Moisture Content":dbl)  [unwired: 3 in, 1 out]
            }
            frame "&HeatVal" {
              n73 = Fract/Exp String To Number(string=w224) -> (number=→"Heating Val":dbl)  [unwired: 3 in, 1 out]
            }
            frame "&InitialWeight" {
              n74 = Fract/Exp String To Number(string=w226) -> (number=→"Measured IMC":dbl)  [unwired: 3 in, 1 out]
            }
            frame "&MTDryer" {
              n75 = Fract/Exp String To Number(string=w228) -> (number=→"Empty Dryer Wt":dbl)  [unwired: 3 in, 1 out]
            }
          }
          n76 = Search and Replace String(input string=w215, search string=w209, replace string=w208) -> (result string=w210:string)  [unwired: 5 in, 3 out]
        }
        n77 = Spreadsheet String To Array(format string=w204, spreadsheet string=w203, array type (2D Dbl)=w204) -> (array=w191:string[][])  [unwired: 1 in]
        n78 = Bundle By Name(cluster=w194, "File Data Out"=w191) -> (w193:T6)
        n79 = local write "File Data Out"(w191) -> ()
        n80 = call <vilib>:"Add State(s) to Queue__jki_lib_state_machine.vi"("State(s) in (\"\")"=w207) -> ("States Out"=w206:string)  [unwired: 14 in]
      }
      frame "Get Final Data" {
        w241 = 1  # column index
        w252 = "" ("format string")
        # "Your code here.\n(You can make a copy of, or modify, this frame)"
        n81 = Unbundle By Name(w257) -> ("File Data Out"=w243:string[][], "File Data In"=w232:string[][])
        n82 = Array Size(array=w232) -> (size(s)=w249:i32[])
        n83 = Index Array(array=w249, index=0) -> (element=w242:i32)
        n84 = Increment(x=w241) -> (x+1=w231:i32)
        n85 = Array Subset(array=w232, index (row)=0 ("index"), length (row)=w242, index (col)=w241, length (col)=1 ("length")) -> (w247:string[][])
        n86 = local read "BDW"() -> (w237:dbl)
        n87 = Reshape Array(w247, w242) -> (w244:string[])
        n88 = Search 1D Array(1D array=w244, element="Final Weight:" ("Delimiter")) -> (index of element=w230:i32)  [unwired: 1 in]
        n89 = Index Array(array=w232, index (row)=w230, index (col)=w231) -> (element=w239:string)
        n90 = Fract/Exp String To Number(string=w239) -> (number=w238:dbl)  [unwired: 3 in, 1 out]
        "FMC (lbs)" <- w238
        n91 = Divide(x=w238, y=w237) -> (x/y=w236:dbl)
        n92 = Decrement(x=w236) -> (x-1=w235:dbl)
        n93 = Multiply(x=w235, y=100.0) -> (x*y=w229:dbl)
        "Final Moisture %" <- w229
        "FMC %" <- w229
        n94 = Number To Fractional String(number=w229) -> (F-format string=w233:string)  [unwired: 3 in]
        n95 = Bundle("String"=w239, w233) -> (w261:cluster{"String":string, string})  [unwired: 1 in]
        n96 = Cluster To Array(cluster=w261) -> (array=w240:string[])
        n97 = call "String2Array.vi"("Delimiter"="\\n", "String"="&FinalWeight\n&FMC") -> ("Array"=w260:string[])  [unwired: 9 in]
        n98 = Array To Spreadsheet String(array=w243, 3:"" ("format string")) -> (spreadsheet string=w254:string)  [unwired: 1 in]
        n99 = for {
          tunnel: w260 -> [w266] mode=indexing
          shift-right: [w267] -> w255
          shift-left: w254 -> [w268]
          tunnel: w240 -> [w265] mode=indexing
          n100 = Search and Replace String(input string=w268, search string=w266, replace string=w265) -> (result string=w267:string)  [unwired: 5 in, 3 out]
        }
        n101 = Spreadsheet String To Array(format string=w252, spreadsheet string=w255, array type (2D Dbl)=w252) -> (array=w251:string[][])  [unwired: 1 in]
        n102 = Bundle By Name(cluster=w257, "File Data Out"=w251) -> (w256:T6)
        n103 = local write "File Data Out"(w251) -> ()
        n104 = call <vilib>:"Add State(s) to Queue__jki_lib_state_machine.vi"("State(s) in (\"\")"=w264) -> ("States Out"=w263:string)  [unwired: 14 in]
      }
      frame "Parse Logged Data" {
        # "Add the data after the header"
        # "Your code here.\n(You can make a copy of, or modify, this frame)"
        n105 = global read "Global Test Variables DPT.vi" "Header Search Key2"() -> (w270:string)
        n106 = global read "Global Test Variables DPT.vi" "Header Search Key1"() -> (w271:string)
        n107 = Unbundle By Name(w282) -> ("File Data In"=w277:string[][])
        n108 = Index Array(array=w277, index (col)=0 ("disabled index (col)")) -> (element=w269:string[])  [unwired: 1 in]
        n109 = Search 1D Array(1D array=w269, element=w271) -> (index of element=w274:i32)  [unwired: 1 in]
        n110 = Search 1D Array(1D array=w269, element=w270) -> (index of element=w273:i32)  [unwired: 1 in]
        n111 = Greater Than 0?(x=w274) -> (x > 0?=w275:bool)
        n112 = Greater Than 0?(x=w273) -> (x > 0?=w278:bool)
        n113 = disable-structure shown="Enabled" {
          disable-tunnel: [w288 w289] -> w279
          disable-tunnel: w278 -> [w287 _]
          disable-tunnel: w275 -> [w286 w289]
          frame Disabled {
            n114 = Exclusive Or(1:w287, 2:w286) -> (0:w288:bool)
          }
          frame Enabled {
          }
        }
        n115 = Select(t=w274, s=w275, f=w273) -> (s? t:f=w272:i32)
        n116 = case shown="True" w279 {
          tunnel: w282 -> [w293 w327]
          tunnel: [w292 w326] -> w281
          tunnel: w277 -> [w291 w325]
          tunnel: ["Macro: Exit" ("element") _] -> w276
          tunnel: w272 -> [_ w323]
          frame False {
            n117 = Bundle By Name(cluster=w293, "File Data Out"=w291) -> (w292:T6)
          }
          frame True {
            w304 = 0 ("index")
            w311 = TRUE
            w303 = 1 ("index")
            # "Delete Columns with Empty Header"
            # "remove end data\nwhere I< on. MSG lines\ngive 0."
            # "Add only the dryer on data.  Dryer is on when \nIL1 > min current (0.1A)"
            n118 = Delete From Array(array=w325, length=w323, index (row)=0) -> (array with subset deleted=w320:string[][])  [unwired: 1 in, 1 out]
            n119 = global read "Global Test Variables DPT.vi" "Dryer On Min Current"() -> (w297:dbl)
            n120 = Delete From Array(array=w320, index (row)=0) -> (deleted portion=w294:string[], array with subset deleted=w301:string[][])  [unwired: 2 in]
            n121 = global read "Global Test Variables DPT.vi" "IL1 Header"() -> (w318:string)
            n122 = global read "Global Test Variables DPT.vi" "IL2 Header"() -> (w307:string)
            n123 = Search 1D Array(1D array=w294, element=w318) -> (index of element=w317:i32)  [unwired: 1 in]
            n124 = Array Subset(array=w301, index (row)=w304, index (col)=w317, length (col)=w303) -> (w316:string[][])  [unwired: 1 in]
            n125 = Array Size(array=w316) -> (size(s)=w321:i32[])
            n126 = Multiply Array Elements(1:w321) -> (0:w300:i32)
            n127 = Reshape Array(w316, w300) -> (w322:string[])
            n128 = Fract/Exp String To Number(string=w322) -> (number=w299:dbl[])  [unwired: 3 in, 1 out]
            n129 = Search 1D Array(1D array=w294, element=w307) -> (index of element=w302:i32)  [unwired: 1 in]
            n130 = Array Subset(array=w301, index (row)=w304, index (col)=w302, length (col)=w303) -> (w306:string[][])  [unwired: 1 in]
            n131 = Reshape Array(w306, w300) -> (w305:string[])
            n132 = Fract/Exp String To Number(string=w305) -> (number=w298:dbl[])  [unwired: 3 in, 1 out]
            n133 = Add(x=w299, y=w298) -> (x+y=w296:dbl[])
            n134 = Greater?(x=w296, y=w297) -> (0:w313:bool[])
            n135 = Reverse 1D Array(array=w313) -> (reversed array=w312:bool[])
            n136 = Search 1D Array(1D array=w313, element=w311) -> (index of element=w315:i32)  [unwired: 1 in]
            n137 = Search 1D Array(1D array=w312, element=w311) -> (index of element=w309:i32)  [unwired: 1 in]
            n138 = Subtract(x=w300, y=w315) -> (x-y=w310:i32)
            n139 = Subtract(x=w310, y=w309) -> (x-y=w308:i32)
            n140 = Array Subset(array=w301, index (row)=w315, length (row)=w308) -> (w295:string[][])  [unwired: 2 in]
            n141 = Fract/Exp String To Number(string=w295) -> (number=w314:dbl[][])  [unwired: 3 in, 1 out]
            n142 = Bundle By Name(cluster=w327, "Header Labels"=w294, "Data"=w314) -> (w326:T6)
          }
        }
        n143 = call <vilib>:"Add State(s) to Queue__jki_lib_state_machine.vi"("State(s) in Front (\"\")"=w276, "State(s) in (\"\")"=w285) -> ("States Out"=w284:string)  [unwired: 13 in]
      }
      frame "Parse Weight Data" {
        w372 = 60.0  # sec/min
        w347 = 0 ("index")
        w341 = 1 ("index")
        # "Just data"
        # "Add the data after the header"
        # "Your code here.\n(You can make a copy of, or modify, this frame)"
        n144 = global read "Global Test Variables DPT.vi" "Header Search Key2"() -> (w390:string)
        n145 = global read "Global Test Variables DPT.vi" "Header Search Key1"() -> (w391:string)
        n146 = Unbundle By Name(w365) -> ("File Data In"=w396:string[][])
        n147 = Index Array(array=w396, index (col)=0 ("disabled index (col)")) -> (element=w389:string[])  [unwired: 1 in]
        n148 = for {
          tunnel: string[] ["Raw Weight", "Weight", "Corrected Weight", "End Weight", "Start Weight"] -> [w413] mode=indexing
          tunnel: [w412] -> w337
          i -> [w411]
          n149 = global read "Global Test Variables DPT.vi" "Time Header"() -> (w412:string)
          n150 = property on="Weight/Raw Weight Data" class="XYGraph (strict)"("Plot.Plot Name"=w413, "Active Plot"=w411, "Value"=T2 [] ("Weight/Raw Weight Data")) -> ()  [unwired: 2 in, 2 out]
        }
        n151 = Search 1D Array(1D array=w389, element=w391) -> (index of element=w394:i32)  [unwired: 1 in]
        n152 = Search 1D Array(1D array=w389, element=w390) -> (index of element=w393:i32)  [unwired: 1 in]
        n153 = Greater Than 0?(x=w394) -> (x > 0?=w395:bool)
        n154 = global read "Global Test Variables DPT.vi" "Corrected Weight Header"() -> (w352:string)
        n155 = Select(t=w394, s=w395, f=w393) -> (s? t:f=w392:i32)
        n156 = global read "Global Test Variables DPT.vi" "Raw Weight Header"() -> (w383:string)
        n157 = global read "Global Test Variables DPT.vi" "Weight Header"() -> (w380:string)
        n158 = Delete From Array(array=w396, length=w392, index (row)=0) -> (array with subset deleted=w385:string[][])  [unwired: 1 in, 1 out]
        n159 = local read "Empty Dryer Wt"() -> (w356:dbl)
        n160 = local read "Measured IMC"() -> (w360:dbl)
        n161 = Delete From Array(array=w385, index (row)=0) -> (deleted portion=w351:string[], array with subset deleted=w348:string[][])  [unwired: 2 in]
        n162 = local read "FMC (lbs)"() -> (w357:dbl)
        n163 = Search 1D Array(1D array=w351, element=w352) -> (index of element=w342:i32)  [unwired: 1 in]
        n164 = Search 1D Array(1D array=w351, element=w337) -> (index of element=w375:i32)  [unwired: 1 in]
        n165 = Search 1D Array(1D array=w351, element=w383) -> (index of element=w382:i32)  [unwired: 1 in]
        n166 = Search 1D Array(1D array=w351, element=w380) -> (index of element=w377:i32)  [unwired: 1 in]
        n167 = Add(x=w356, y=w357) -> (x+y=w333:dbl)
        n168 = Add(x=w356, y=w360) -> (x+y=w331:dbl)
        n169 = Array Subset(array=w348, index (row)=w347, index (col)=w375, length (col)=w341) -> (w374:string[][])  [unwired: 1 in]
        n170 = Array Subset(array=w348, index (row)=w347, index (col)=w382, length (col)=w341) -> (w381:string[][])  [unwired: 1 in]
        n171 = Array Subset(array=w348, index (row)=w347, index (col)=w377, length (col)=w341) -> (w379:string[][])  [unwired: 1 in]
        n172 = Array Subset(array=w348, index (row)=w347, index (col)=w342, length (col)=w341) -> (w343:string[][])  [unwired: 1 in]
        n173 = Array Size(array=w381) -> (size(s)=w386:i32[])
        n174 = Multiply Array Elements(1:w386) -> (0:w344:i32)
        n175 = Reshape Array(w374, w344) -> (w373:string[])
        n176 = Fract/Exp String To Number(string=w373, default (0 dbl)=w372) -> (number=w371:dbl[])  [unwired: 2 in, 1 out]
        n177 = Reshape Array(w343, w344) -> (w346:string[])
        n178 = Reshape Array(w379, w344) -> (w378:string[])
        n179 = Reshape Array(w381, w344) -> (w387:string[])
        n180 = local read "Empty Dryer Wt"() -> (w339:dbl)
        n181 = Index Array(array=w371, index=0) -> (element=w345:dbl)
        n182 = flat-sequence {
          tunnel: w370 -> [w409]
          tunnel: [2.0 ("x")] -> w336
          frame #0 {
            "Weight/Raw Weight Data" <- w409
          }
        }
        n183 = Fract/Exp String To Number(string=w387) -> (number=w367:dbl[])  [unwired: 3 in, 1 out]
        n184 = Fract/Exp String To Number(string=w346) -> (number=w329:dbl[])  [unwired: 3 in, 1 out]
        n185 = Fract/Exp String To Number(string=w378) -> (number=w366:dbl[])  [unwired: 3 in, 1 out]
        n186 = while {
          shift-right: [w403] -> _
          shift-left: w329 -> [w407]
          tunnel: [w401] -> w328
          stop <- w402 stop-if-true
          n187 = Delete From Array(array=w407, length=1) -> (deleted portion=w405:dbl[], array with subset deleted=w403:dbl[])  [unwired: 1 in]
          n188 = Index Array(array=w405, index=0) -> (element=w401:dbl)
          n189 = Greater Than 0?(x=w401) -> (x > 0?=w402:bool)
        }
        "FMC (lbs) Predicted" <- w328
        n190 = Add(x=w339, y=w329) -> (x+y=w340:dbl[])
        n191 = Subtract(x=w371, y=w345) -> (x-y=w361:dbl[])
        n192 = Divide(x=w361, y=w372) -> (x/y=w330:dbl[])
        n193 = Less Than 0?(x=w330) -> (x < 0?=w364:bool[])
        n194 = Array Size(array=w330) -> (size(s)=w355:i32)
        n195 = Initialize Array(w331, w355) -> (w359:dbl[])
        n196 = Initialize Array(w333, w355) -> (w353:dbl[])
        n197 = Search 1D Array(1D array=w364, element=TRUE) -> (index of element=w362:i32)  [unwired: 1 in]
        n198 = Add(x=w336, y=w331) -> (x+y=w334:dbl)
        n199 = Add(x=-2.0, y=w333) -> (x+y=w332:dbl)
        n200 = case shown="0, Default" w362 {
          selector: w362 -> [w416 _]
          tunnel: w330 -> [w419 w420]
          tunnel: w362 -> [w418 _]
          tunnel: w355 -> [w415 _]
          tunnel: [w414 w420] -> w349
          frame 0, Default {
            n201 = Subtract(x=w415, y=w416) -> (x-y=w417:i32)
            n202 = Delete From Array(array=w419, length=w417, index=w418) -> (array with subset deleted=w414:dbl[])  [unwired: 1 out]
          }
          frame -1 {
          }
        }
        n203 = Bundle(w349, w340) -> (w350:cluster{dbl[], dbl[]})  [unwired: 1 in]
        n204 = Bundle(w349, w367) -> (w368:cluster{dbl[], dbl[]})  [unwired: 1 in]
        n205 = Bundle(w349, w359) -> (w358:cluster{dbl[], dbl[]})  [unwired: 1 in]
        n206 = Bundle(w349, w353) -> (w354:cluster{dbl[], dbl[]})  [unwired: 1 in]
        n207 = Bundle(w349, w366) -> (w369:cluster{dbl[], dbl[]})  [unwired: 1 in]
        n208 = Build Array(w369, w368, w350, w358, w354) -> (w370:cluster{dbl[], dbl[]}[])
        n209 = property on="Weight/Raw Weight Data" class="XYGraph (strict)"("YScale.Maximum"=w334, "YScale.Minimum"=w332) -> ()  [unwired: 2 in, 2 out]
        n210 = call <vilib>:"Add State(s) to Queue__jki_lib_state_machine.vi"("State(s) in (\"\")"=w400) -> ("States Out"=w399:string)  [unwired: 14 in]
      }
      frame "Remove Empty Data" {
        # "These are the elements in column 0 to indicate where\nthe header for the data is."
        # "Your code here.\n(You can make a copy of, or modify, this frame)"
        n211 = Unbundle By Name(w425) -> ("Data"=w428:dbl[][], "Header Labels"=w429:string[])
        n212 = Transpose 2D Array(2D array=w428) -> (transposed array=w427:dbl[][])
        n213 = for {
          tunnel: w429 -> [w437] mode=indexing
          shift-right: [w438] -> w421
          shift-left: string[] [] ("deleted portion") -> [w439]
          tunnel: w427 -> [w434] mode=indexing
          shift-right: [w435] -> w423
          shift-left: dbl[][] [] ("number") -> [w436]
          n214 = Equal?(x=w437, y="") -> (x = y?=w440:bool)
          n215 = case shown="True" w440 {
            tunnel: [w446 w449] -> w438
            tunnel: w439 -> [w447 w449]
            tunnel: w437 -> [w445 _]
            tunnel: w436 -> [w444 w448]
            tunnel: [w443 w448] -> w435
            tunnel: w434 -> [w442 _]
            frame False {
              n216 = Build Array (concatenate)(w447, w445) -> (w446:string[])
              n217 = Build Array (concatenate)(w444, w442) -> (w443:dbl[][])
            }
            frame True {
            }
          }
        }
        "Header" <- w421
        n218 = Transpose 2D Array(2D array=w423) -> (transposed array=w422:dbl[][])
        n219 = Bundle By Name(cluster=w425, "Data"=w422, "Header Labels"=w421) -> (w424:T6)
        n220 = call <vilib>:"Add State(s) to Queue__jki_lib_state_machine.vi"("State(s) in (\"\")"=w433) -> ("States Out"=w432:string)  [unwired: 14 in]
      }
      frame "Insert VL1 MaxMin" {
        w454 = "&VL1MaxMin"  # replacement term
        w470 = i16 1 ("precision (6)")
        # "column of term"
        # "These are the elements in column 0 to indicate where\nthe header for the data is."
        # "Your code here.\n(You can make a copy of, or modify, this frame)"
        n221 = Unbundle By Name(w457) -> ("Data"=w459:dbl[][], "Header Labels"=w461:string[])
        n222 = global read "Global Test Variables DPT.vi" "VL1 Header"() -> (w464:string)
        n223 = Array Size(array=w459) -> (size(s)=w472:i32[])
        n224 = Search 1D Array(1D array=w461, element=w464) -> (index of element=w463:i32)  [unwired: 1 in]
        n225 = Index Array(array=w472, index=0) -> (element=w460:i32)
        n226 = Array Subset(array=w459, length (row)=w460, index (col)=w463, length (col)=1 ("length")) -> (w458:dbl[][])  [unwired: 1 in]
        n227 = Array Max & Min(array=w458) -> (max value=w466:dbl, min value=w465:dbl)  [unwired: 2 out]
        n228 = Number To Fractional String(number=w466, precision (6)=w470) -> (F-format string=w469:string)  [unwired: 2 in]
        n229 = Number To Fractional String(number=w465, precision (6)=w470) -> (F-format string=w467:string)  [unwired: 2 in]
        n230 = Concatenate Strings(w469, "/" ("string"), w467) -> (w451:string)
        n231 = Search and Replace String(input string="Replace Data Out Term >> xxx,yyy" ("State(s) in Front (\"\")"), search string="xxx", replace string=w454) -> (result string=w452:string)  [unwired: 5 in, 3 out]
        n232 = Search and Replace String(input string=w452, search string="yyy", replace string=w451) -> (result string=w450:string)  [unwired: 5 in, 3 out]
        n233 = call <vilib>:"Add State(s) to Queue__jki_lib_state_machine.vi"("State(s) in Front (\"\")"=w450, "State(s) in (\"\")"=w475) -> ("States Out"=w474:string)  [unwired: 13 in]
      }
      frame "Insert VL2 MaxMin" {
        w480 = "&VL2MaxMin"  # replacement term
        w496 = i16 1 ("precision (6)")
        # "column of term"
        # "These are the elements in column 0 to indicate where\nthe header for the data is."
        # "Your code here.\n(You can make a copy of, or modify, this frame)"
        n234 = Unbundle By Name(w483) -> ("Data"=w485:dbl[][], "Header Labels"=w487:string[])
        n235 = global read "Global Test Variables DPT.vi" "VL2 Header"() -> (w490:string)
        n236 = Array Size(array=w485) -> (size(s)=w498:i32[])
        n237 = Search 1D Array(1D array=w487, element=w490) -> (index of element=w489:i32)  [unwired: 1 in]
        n238 = Index Array(array=w498, index=0) -> (element=w486:i32)
        n239 = Array Subset(array=w485, length (row)=w486, index (col)=w489, length (col)=1 ("length")) -> (w484:dbl[][])  [unwired: 1 in]
        n240 = Array Max & Min(array=w484) -> (max value=w492:dbl, min value=w491:dbl)  [unwired: 2 out]
        n241 = Number To Fractional String(number=w492, precision (6)=w496) -> (F-format string=w495:string)  [unwired: 2 in]
        n242 = Number To Fractional String(number=w491, precision (6)=w496) -> (F-format string=w493:string)  [unwired: 2 in]
        n243 = Concatenate Strings(w495, "/" ("string"), w493) -> (w477:string)
        n244 = Search and Replace String(input string="Replace Data Out Term >> xxx,yyy" ("State(s) in Front (\"\")"), search string="xxx", replace string=w480) -> (result string=w478:string)  [unwired: 5 in, 3 out]
        n245 = Search and Replace String(input string=w478, search string="yyy", replace string=w477) -> (result string=w476:string)  [unwired: 5 in, 3 out]
        n246 = call <vilib>:"Add State(s) to Queue__jki_lib_state_machine.vi"("State(s) in Front (\"\")"=w476, "State(s) in (\"\")"=w501) -> ("States Out"=w500:string)  [unwired: 13 in]
      }
      frame "Insert Tamb MaxMin" {
        w506 = "&TempMaxMin"  # replacement term
        w522 = i16 1 ("precision (6)")
        # "column of term"
        # "These are the elements in column 0 to indicate where\nthe header for the data is."
        # "Your code here.\n(You can make a copy of, or modify, this frame)"
        n247 = Unbundle By Name(w509) -> ("Data"=w511:dbl[][], "Header Labels"=w513:string[])
        n248 = global read "Global Test Variables DPT.vi" "Tambient Header"() -> (w516:string)
        n249 = Array Size(array=w511) -> (size(s)=w524:i32[])
        n250 = Search 1D Array(1D array=w513, element=w516) -> (index of element=w515:i32)  [unwired: 1 in]
        n251 = Index Array(array=w524, index=0) -> (element=w512:i32)
        n252 = Array Subset(array=w511, length (row)=w512, index (col)=w515, length (col)=1 ("length")) -> (w510:dbl[][])  [unwired: 1 in]
        n253 = Array Max & Min(array=w510) -> (max value=w518:dbl, min value=w517:dbl)  [unwired: 2 out]
        n254 = Number To Fractional String(number=w518, precision (6)=w522) -> (F-format string=w521:string)  [unwired: 2 in]
        n255 = Number To Fractional String(number=w517, precision (6)=w522) -> (F-format string=w519:string)  [unwired: 2 in]
        n256 = Concatenate Strings(w521, "/" ("string"), w519) -> (w503:string)
        n257 = Search and Replace String(input string="Replace Data Out Term >> xxx,yyy" ("State(s) in Front (\"\")"), search string="xxx", replace string=w506) -> (result string=w504:string)  [unwired: 5 in, 3 out]
        n258 = Search and Replace String(input string=w504, search string="yyy", replace string=w503) -> (result string=w502:string)  [unwired: 5 in, 3 out]
        n259 = call <vilib>:"Add State(s) to Queue__jki_lib_state_machine.vi"("State(s) in Front (\"\")"=w502, "State(s) in (\"\")"=w527) -> ("States Out"=w526:string)  [unwired: 13 in]
      }
      frame "Insert RH MaxMin" {
        w532 = "&RHMaxMin"  # replacement term
        w548 = i16 1 ("precision (6)")
        # "column of term"
        # "These are the elements in column 0 to indicate where\nthe header for the data is."
        # "Your code here.\n(You can make a copy of, or modify, this frame)"
        n260 = Unbundle By Name(w535) -> ("Data"=w537:dbl[][], "Header Labels"=w539:string[])
        n261 = global read "Global Test Variables DPT.vi" "RH Header"() -> (w542:string)
        n262 = Array Size(array=w537) -> (size(s)=w550:i32[])
        n263 = Search 1D Array(1D array=w539, element=w542) -> (index of element=w541:i32)  [unwired: 1 in]
        n264 = Index Array(array=w550, index=0) -> (element=w538:i32)
        n265 = Array Subset(array=w537, length (row)=w538, index (col)=w541, length (col)=1 ("length")) -> (w536:dbl[][])  [unwired: 1 in]
        n266 = Array Max & Min(array=w536) -> (max value=w544:dbl, min value=w543:dbl)  [unwired: 2 out]
        n267 = Number To Fractional String(number=w544, precision (6)=w548) -> (F-format string=w547:string)  [unwired: 2 in]
        n268 = Number To Fractional String(number=w543, precision (6)=w548) -> (F-format string=w545:string)  [unwired: 2 in]
        n269 = Concatenate Strings(w547, "/" ("string"), w545) -> (w529:string)
        n270 = Search and Replace String(input string="Replace Data Out Term >> xxx,yyy" ("State(s) in Front (\"\")"), search string="xxx", replace string=w532) -> (result string=w530:string)  [unwired: 5 in, 3 out]
        n271 = Search and Replace String(input string=w530, search string="yyy", replace string=w529) -> (result string=w528:string)  [unwired: 5 in, 3 out]
        n272 = call <vilib>:"Add State(s) to Queue__jki_lib_state_machine.vi"("State(s) in Front (\"\")"=w528, "State(s) in (\"\")"=w553) -> ("States Out"=w552:string)  [unwired: 13 in]
      }
      frame "Reformat Date" {
        w563 = "-"
        w568 = 1  # column of Date Data
        # "Fixme: Need Seconds if debug log is way off!"
        # "These are the elements in column 0 to indicate where\nthe header for the data is."
        # "Your code here.\n(You can make a copy of, or modify, this frame)"
        n273 = Unbundle By Name(w556) -> ("File Data Out"=w570:string[][])
        n274 = Index Array(array=w570, index (col)=0 ("disabled index (col)")) -> (element=w554:string[])  [unwired: 1 in]
        n275 = global read "Global Test Variables DPT.vi" "Date Label"() -> (w571:string)
        n276 = Search 1D Array(1D array=w554, element=w571) -> (index of element=w569:i32)  [unwired: 1 in]
        n277 = Index Array(array=w570, index (row)=w569, index (col)=w568) -> (element=w566:string)
        n278 = Scan From String(format string="%4s%2s%2s%3s%2s", input string=w566) -> (output 1=w565:string, output 2=w564:string, output 3=w561:string, output 4=w560:string, output 5=w559:string)  [unwired: 7 in, 3 out]
        n279 = Concatenate Strings(w565, w563, w564, w563, w561, w560, ":" ("string"), w559) -> (w558:string)
        "Date String" <- w558
        n280 = Replace Array Subset(array=w570, new element=w558, index (row)=w569, index (col)=w568) -> (w555:string[][])
        n281 = Bundle By Name(cluster=w556, "File Data Out"=w555) -> (w557:T6)
        n282 = call <vilib>:"Add State(s) to Queue__jki_lib_state_machine.vi"("State(s) in (\"\")"=w575) -> ("States Out"=w574:string)  [unwired: 14 in]
      }
      frame "Frequency Check" {
        w583 = 1  # column of freq Data
        # "These are the elements in column 0 to indicate where\nthe header for the data is."
        # "Your code here.\n(You can make a copy of, or modify, this frame)"
        n283 = Unbundle By Name(w581) -> ("File Data Out"=w584:string[][])
        n284 = Index Array(array=w584, index (col)=0 ("disabled index (col)")) -> (element=w586:string[])  [unwired: 1 in]
        n285 = global read "Global Test Variables DPT.vi" "Frequency Label"() -> (w585:string)
        n286 = Search 1D Array(1D array=w586, element=w585) -> (index of element=w579:i32)  [unwired: 1 in]
        n287 = Index Array(array=w584, index (row)=w579, index (col)=w583) -> (element=w578:string)
        n288 = Equal?(x=w578, y="") -> (x = y?=w576:bool)
        n289 = case shown="False" w576 {
          tunnel: w584 -> [w591 w596]
          tunnel: w583 -> [_ w595]
          tunnel: [w591 w594] -> w580
          tunnel: w579 -> [_ w593]
          frame False {
          }
          frame True {
            n290 = Replace Array Subset(array=w596, new element="60" ("new element/subarray"), index (row)=w593, index (col)=w595) -> (w594:string[][])
          }
        }
        n291 = Bundle By Name(cluster=w581, "File Data Out"=w580) -> (w582:T6)
        n292 = call <vilib>:"Add State(s) to Queue__jki_lib_state_machine.vi"("State(s) in (\"\")"=w590) -> ("States Out"=w589:string)  [unwired: 14 in]
      }
      frame "Insert RMC Corrected" {
        w612 = 180  # MA half size
        w617 = 0.01  # Steady Weight Threshold
        w618 = 0.0
        w631 = 60.0  # Sec per Min
        w660 = 40  # Initial MC taken from 40 samples In
        # "Time"
        # "RMC Cor"
        # "column of term"
        # "These are the elements in column 0 to indicate where\nthe header for the data is."
        # "Your code here.\n(You can make a copy of, or modify, this frame)"
        n293 = Unbundle By Name(w648) -> ("Data"=w619:dbl[][], "Header Labels"=w621:string[])
        n294 = global read "Global Test Variables DPT.vi" "RMC Header"() -> (w661:string)
        n295 = global read "Global Test Variables DPT.vi" "Time Header"() -> (w641:string)
        n296 = Search 1D Array(1D array=w621, element=w641) -> (index of element=w642:i32)  [unwired: 1 in]
        n297 = Search 1D Array(1D array=w621, element=w661) -> (index of element=w650:i32)  [unwired: 1 in]
        n298 = Search 1D Array(1D array=w621, element="Corrected Weight") -> (index of element=w622:i32)  [unwired: 1 in]
        n299 = call "Array-Get 1D Column fr 2D.vi"("2D Array Data"=w619, "column index"=w650) -> ("Column Data"=w651:dbl[])  [unwired: 13 in]
        n300 = call "Array-Get 1D Column fr 2D.vi"("2D Array Data"=w619, "column index"=w642) -> ("Column Data"=w635:dbl[])  [unwired: 13 in]
        n301 = call "Array-Get 1D Column fr 2D.vi"("2D Array Data"=w619, "column index"=w622) -> ("Column Data"=w614:dbl[])  [unwired: 13 in]
        n302 = local read "Init Moisture Content"() -> (w658:dbl)
        n303 = local read "Final Moisture %"() -> (w657:dbl)
        n304 = Array Size(array=w651) -> (size(s)=w659:i32)
        n305 = Index Array(array=w635, index=0) -> (element=w634:dbl)
        n306 = for {
          tunnel: w614 -> [w671] mode=indexing
          shift-right: [w671] -> _
          shift-left: w618 -> [_]
          shift-left: w618 -> [w670]
          tunnel: w617 -> [w667]
          tunnel: [w665] -> w609
          i -> [w665]
          stop <- w666 stop-if-true
          n307 = Subtract(x=w671, y=w670) -> (x-y=w669:dbl)
          n308 = Absolute Value(x=w669) -> (abs(x)=w668:dbl)
          n309 = Less?(x=w668, y=w667) -> (x < y?=w666:bool)
        }
        n310 = Decrement(x=w659) -> (x-1=w644:i32)
        n311 = Increment(x=w650) -> (x+1=w643:i32)
        n312 = Subtract(x=w635, y=w634) -> (x-y=w632:dbl[])
        n313 = Index Array(array=w651, index #1=w660, index #2=w644) -> (element #1=w654:dbl, element #2=w653:dbl)
        n314 = Divide(x=w632, y=w631) -> (x/y=w630:dbl[])
        n315 = Bundle(w654, w653) -> (w655:cluster{dbl, dbl})  [unwired: 1 in]
        n316 = Bundle("Init Moisture Content"=w658, "Final Moisture %"=w657) -> (w656:T8)  [unwired: 1 in]
        n317 = Cluster To Array(cluster=w655) -> (array=w652:dbl[])
        n318 = Cluster To Array(cluster=w656) -> (array=w601:dbl[])
        n319 = Delete From Array(array=w614, length=w609, index=0) -> (deleted portion=w610:dbl[], array with subset deleted=w613:dbl[])
        n320 = call <vilib>:"Interpolate 1D.vi"("xi"=w651, "X"=w652, "Y"=w601) -> ("yi"=w599:dbl[])  [unwired: 6 in, 2 out]
        n321 = Add(x=w609, y=5) -> (x+y=w607:i32)
        n322 = call "Moving Average Half Center.vi"("MA half size"=w612, "Data Array"=w613) -> ("Moving Average"=w611:dbl[])  [unwired: 9 in]
        n323 = Array Max & Min(array=w630) -> (max value=w628:dbl)  [unwired: 3 out]
        n324 = Build Array (concatenate)(w610, w611) -> (w600:dbl[])
        n325 = Insert Into Array(array=w621, index=w643, new element #1="RMC Corrected" ("new element/subarray"), new element #2="RMC(Wf)" ("new element/subarray")) -> (w645:string[])
        n326 = Array Size(array=w600) -> (size(s)=w606:i32)
        n327 = Decrement(x=w606) -> (x-1=w597:i32)
        n328 = Index Array(array=w600, index #1=w607, index #2=w597) -> (element #1=w604:dbl, element #2=w603:dbl)
        n329 = Bundle("mean"=w604, "mean"=w603) -> (w605:cluster{"mean":dbl, "mean":dbl})  [unwired: 1 in]
        n330 = Cluster To Array(cluster=w605) -> (array=w602:dbl[])
        n331 = call <vilib>:"Interpolate 1D.vi"("xi"=w600, "X"=w602, "Y"=w601) -> ("yi"=w598:dbl[])  [unwired: 6 in, 2 out]
        n332 = call <vilib>:"Interpolate 1D.vi"("xi"=dbl[] [3.0, 4.0, 5.0] ("Column Data"), "X"=w598, "Y"=w630) -> ("yi"=w629:dbl[])  [unwired: 6 in, 2 out]
        n333 = Insert Into Array(array=w619, index (col)=w643, new element #1=w599, new element #2=w598) -> (w646:dbl[][])  [unwired: 1 in]
        n334 = Bundle By Name(cluster=w648, "Data"=w646, "Header Labels"=w645) -> (w647:T6)
        n335 = Array To Cluster(array=w629) -> (cluster=w639:cluster{"yi[0]":dbl, "yi[1]":dbl, "yi[2]":dbl})
        n336 = Greater?(x=w629, y=w628) -> (0:w626:bool[])
        n337 = Unbundle(w639) -> ("yi[0]"=→"TT 3%":dbl, "yi[1]"=→"TT 4%":dbl, "yi[2]"=→"TT 5%":dbl)
        n338 = Array To Cluster(array=w626) -> (cluster=w627:cluster{"[0]":bool, "[1]":bool, "[2]":bool})
        n339 = Unbundle(w627) -> ("[0]"=→"TT3 Extrapolated":bool, "[1]"=→"TT4 Extrapolated":bool, "[2]"=→"TT5 Extrapolated":bool)
        n340 = call <vilib>:"Add State(s) to Queue__jki_lib_state_machine.vi"("State(s) in (\"\")"=w664) -> ("States Out"=w663:string)  [unwired: 14 in]
      }
      frame "Insert Time To Percents" {
        w678 = "&TT3"  # replacement term
        w683 = "&TT4"  # replacement term
        w694 = "&TT5"  # replacement term
        # "These are the elements in column 0 to indicate where\nthe header for the data is."
        # "Your code here.\n(You can make a copy of, or modify, this frame)"
        n341 = local read "TT 3%"() -> (w674:dbl)
        n342 = local read "TT 4%"() -> (w687:dbl)
        n343 = local read "TT 5%"() -> (w689:dbl)
        n344 = Number To Fractional String(number=w674) -> (F-format string=w675:string)  [unwired: 3 in]
        n345 = Number To Fractional String(number=w687) -> (F-format string=w686:string)  [unwired: 3 in]
        n346 = Search and Replace String(input string="Replace Data Out Term >> xxx,yyy" ("State(s) in Front (\"\")"), search string="xxx", replace string=w678) -> (result string=w676:string)  [unwired: 5 in, 3 out]
        n347 = Number To Fractional String(number=w689) -> (F-format string=w690:string)  [unwired: 3 in]
        n348 = Search and Replace String(input string="Replace Data Out Term >> xxx,yyy\n" ("State(s) in Front (\"\")"), search string="xxx", replace string=w683) -> (result string=w685:string)  [unwired: 5 in, 3 out]
        n349 = Search and Replace String(input string="Replace Data Out Term >> xxx,yyy\n" ("State(s) in Front (\"\")"), search string="xxx", replace string=w694) -> (result string=w692:string)  [unwired: 5 in, 3 out]
        n350 = Search and Replace String(input string=w676, search string="yyy", replace string=w675) -> (result string=w672:string)  [unwired: 5 in, 3 out]
        n351 = Search and Replace String(input string=w685, search string="yyy", replace string=w686) -> (result string=w673:string)  [unwired: 5 in, 3 out]
        n352 = Search and Replace String(input string=w692, search string="yyy", replace string=w690) -> (result string=w691:string)  [unwired: 5 in, 3 out]
        n353 = Concatenate Strings(w691, w673, w672) -> (w688:string)
        n354 = call <vilib>:"Add State(s) to Queue__jki_lib_state_machine.vi"("State(s) in Front (\"\")"=w688, "State(s) in (\"\")"=w700) -> ("States Out"=w699:string)  [unwired: 13 in]
      }
      frame "Insert Heating Value" {
        w705 = 0 ("index")
        # "Insert Column of heating value"
        n355 = Unbundle By Name(w709) -> ("Data"=w712:dbl[][], "Header Labels"=w704:string[])
        n356 = call "Array-Get 1D Column fr 2D.vi"("2D Array Data"=w712, "column index"=0) -> ("Column Data"=w713:dbl[])  [unwired: 13 in]
        n357 = local read "Heating Val"() -> (w702:dbl)
        n358 = Array Size(array=w713) -> (size(s)=w703:i32)
        n359 = Initialize Array(w702, w703) -> (w701:dbl[])
        n360 = Insert Into Array(array=w704, index=w705, new element="HEAT VALUE (BTU/cuFt @ STP)" ("new element/subarray")) -> (w706:string[])
        n361 = Insert Into Array(array=w712, index (col)=w705, new element=w701) -> (w707:dbl[][])  [unwired: 1 in]
        n362 = Bundle By Name(cluster=w709, "Data"=w707, "Header Labels"=w706) -> (w708:T6)
        n363 = call <vilib>:"Add State(s) to Queue__jki_lib_state_machine.vi"("State(s) in (\"\")"=w716) -> ("States Out"=w715:string)  [unwired: 14 in]
      }
      frame "Rescale WH to kWH" {
        w718 = 1000.0  # kWH/WH
        # "These are the elements in column 0 to indicate where\nthe header for the data is."
        # "Your code here.\n(You can make a copy of, or modify, this frame)"
        n364 = Unbundle By Name(w723) -> ("Data"=w725:dbl[][], "Header Labels"=w724:string[])
        n365 = global read "Global Test Variables DPT.vi" "WattHour Header"() -> (w726:string)
        n366 = Search 1D Array(1D array=w724, element=w726) -> (index of element=w720:i32)  [unwired: 1 in]
        n367 = call "Array-Get 1D Column fr 2D.vi"("2D Array Data"=w725, "column index"=w720) -> ("Column Data"=w719:dbl[])  [unwired: 13 in]
        n368 = Divide(x=w719, y=w718) -> (x/y=w717:dbl[])
        n369 = Replace Array Subset(array=w725, new element=w717, index (col)=w720) -> (w721:dbl[][])  [unwired: 1 in]
        n370 = Bundle By Name(cluster=w723, "Data"=w721) -> (w722:T6)
        n371 = call <vilib>:"Add State(s) to Queue__jki_lib_state_machine.vi"("State(s) in (\"\")"=w729) -> ("States Out"=w728:string)  [unwired: 14 in]
      }
      frame "Insert Energy Vals" {
        w763 = 30.0  # ?
        w742 = 459.67  # F to R?
        w761 = 60.0  # Ref Temp
        # "Gas energy wh"
        # "gas vol"
        # "i:cor vol"
        # "h: gas corr factor"
        # "g"
        # "Your code here.\n(You can make a copy of, or modify, this frame)"
        n372 = global read "Global Test Variables DPT.vi" "Bar. Pressure Header"() -> (w782:string)
        n373 = global read "Global Test Variables DPT.vi" "Gas Temp Header"() -> (w773:string)
        n374 = global read "Global Test Variables DPT.vi" "Time Header"() -> (w748:string)
        n375 = global read "Global Test Variables DPT.vi" "Gas Press Header"() -> (w779:string)
        n376 = Unbundle By Name(w781) -> ("Data"=w747:dbl[][], "Header Labels"=w749:string[])
        n377 = global read "Global Test Variables DPT.vi" "Gas Vol Header"() -> (w775:string)
        n378 = Search 1D Array(1D array=w749, element=w748) -> (index of element=w746:i32)  [unwired: 1 in]
        n379 = Search 1D Array(1D array=w749, element=w782) -> (index of element=w778:i32)  [unwired: 1 in]
        n380 = Search 1D Array(1D array=w749, element=w775) -> (index of element=w776:i32)  [unwired: 1 in]
        n381 = Search 1D Array(1D array=w749, element=w779) -> (index of element=w777:i32)  [unwired: 1 in]
        n382 = Search 1D Array(1D array=w749, element=w773) -> (index of element=w772:i32)  [unwired: 1 in]
        n383 = call "Array-Get 1D Column fr 2D.vi"("2D Array Data"=w747, "column index"=w778) -> ("Column Data"=w769:dbl[])  [unwired: 13 in]
        "Bar.Pres E36" <- w769
        n384 = call "Array-Get 1D Column fr 2D.vi"("2D Array Data"=w747, "column index"=w772) -> ("Column Data"=w755:dbl[])  [unwired: 13 in]
        "Gas Temp E38" <- w755
        n385 = call "Array-Get 1D Column fr 2D.vi"("2D Array Data"=w747, "column index"=w776) -> ("Column Data"=w760:dbl[])  [unwired: 13 in]
        "Gas Vol E42" <- w760
        n386 = call "Array-Get 1D Column fr 2D.vi"("2D Array Data"=w747, "column index"=w746) -> ("Column Data"=w745:dbl[])  [unwired: 13 in]
        n387 = call "Array-Get 1D Column fr 2D.vi"("2D Array Data"=w747, "column index"=w777) -> ("Column Data"=w771:dbl[])  [unwired: 13 in]
        "Gas Pres E37" <- w771
        n388 = Index Array(array=w760, index=0) -> (element=w759:dbl)
        "Gas Vol Init E41" <- w759
        n389 = Subtract(x=w760, y=w759) -> (x-y=w757:dbl[])
        n390 = disable-structure shown="Disabled" {
          frame Disabled {
            n391 = call "Worksheet DOE Audit.vi"() -> ()  [unwired: 8 in, 3 out]
          }
          frame Enabled {
            # "Look for ref on formula, taken from xl spread sheet from Dusty Henderson"
          }
        }
        n392 = Multiply(x=0.0735, y=w771) -> (x*y=w768:dbl[])
        n393 = Add(x=w769, y=w768) -> (x+y=w766:dbl[])
        n394 = Add(x=w742, y=w755) -> (x+y=w764:dbl[])
        n395 = local read "Heating Val"() -> (w750:dbl)
        n396 = Add(x=w761, y=w742) -> (x+y=w767:dbl)
        n397 = Multiply(x=w766, y=w767) -> (x*y=w765:dbl[])
        n398 = Multiply(x=w763, y=w764) -> (x*y=w762:dbl[])
        n399 = Divide(x=w765, y=w762) -> (x/y=w758:dbl[])
        n400 = Divide(x=1.0117, y=3.412) -> (x/y=w752:dbl)
        n401 = Compound Arithmetic op=MULTIPLY(w758, w757) -> (w756:dbl[])
        n402 = Compound Arithmetic op=MULTIPLY(w756, w750, w752) -> (w739:dbl[])
        n403 = call "Convert Gas WH to Watts.vi"("TIME"=w745, "WH"=w739) -> ("Watts"=w743:dbl[])  [unwired: 9 in]
        n404 = Insert Into Array(array=w747, index (col)=0 ("disabled index (col)"), new element=w743) -> (w741:dbl[][])  [unwired: 1 in]
        n405 = Insert Into Array(array=w749, index=0, new element="Watts-G" ("new element/subarray")) -> (w736:string[])
        n406 = Divide(x=w739, y=1000.0 ("x")) -> (x/y=w737:dbl[])
        n407 = Insert Into Array(array=w736, index=0, new element="kWhr-G" ("new element/subarray")) -> (w735:string[])
        n408 = call "Convert to Dynamic Data"("Array"=w743) -> ("Dynamic Data Type"=→"Gas W Data":dynamicdata)  [unwired: 3 in]
        n409 = Insert Into Array(array=w741, index (col)=0 ("index (row)"), new element=w737) -> (w740:dbl[][])  [unwired: 1 in]
        n410 = Bundle By Name(cluster=w781, "Data"=w740, "Header Labels"=w735) -> (w780:T6)
        n411 = call <vilib>:"Add State(s) to Queue__jki_lib_state_machine.vi"("State(s) in (\"\")"=w785) -> ("States Out"=w784:string)  [unwired: 14 in]
      }
      frame "Insert kWH Total" {
        w795 = 0 ("index")
        # "Insert Column of heating value"
        n412 = Unbundle By Name(w799) -> ("Data"=w789:dbl[][], "Header Labels"=w791:string[])
        n413 = global read "Global Test Variables DPT.vi" "WattHour Header"() -> (w794:string)
        n414 = Search 1D Array(1D array=w791, element="kWhr-G" ("new element/subarray")) -> (index of element=w790:i32)  [unwired: 1 in]
        n415 = Search 1D Array(1D array=w791, element=w794) -> (index of element=w793:i32)  [unwired: 1 in]
        n416 = call "Array-Get 1D Column fr 2D.vi"("2D Array Data"=w789, "column index"=w793) -> ("Column Data"=w788:dbl[])  [unwired: 13 in]
        n417 = call "Array-Get 1D Column fr 2D.vi"("2D Array Data"=w789, "column index"=w790) -> ("Column Data"=w787:dbl[])  [unwired: 13 in]
        n418 = Add(x=w788, y=w787) -> (x+y=w786:dbl[])
        n419 = Insert Into Array(array=w791, index=w795, new element="kWhr-TOTAL" ("new element/subarray")) -> (w796:string[])
        n420 = Insert Into Array(array=w789, index (col)=w795, new element=w786) -> (w797:dbl[][])  [unwired: 1 in]
        n421 = Bundle By Name(cluster=w799, "Data"=w797, "Header Labels"=w796) -> (w798:T6)
        n422 = call <vilib>:"Add State(s) to Queue__jki_lib_state_machine.vi"("State(s) in (\"\")"=w803) -> ("States Out"=w802:string)  [unwired: 14 in]
      }
      frame "Rename Headers" {
        w804 = string[][] [["P:Sigma", "Watts-E"], ["RMC", "RMC Raw"], ["Wp:Sigma", "kWHr-E"], ["Urms:Element 1", "V-L1"], ["Urms:Element 2", "V-L2"], ["Irms:Element 1", "I-L1"], ["Irms:Element 2", "I-L2"], ["I +peak:Element 1", "I-PEAK-L1"], ["I +peak:Element 2", "I-PEAK-L2"], ["Gas Feedback", "GAS VOLUME (cuFt)"], ["Gas Pressure", "GAS PRES (inH2O)"], ["Gas Temperature", "GAS TEMP"], ["Barometric Pressure", "BAROMETRIC (inHG)"]]  # Rename From, To
        # "Rename Headers: All but time, which is used in last time/rejoin procedure"
        n423 = Unbundle By Name(w808) -> ("Header Labels"=w805:string[])
        n424 = for {
          tunnel: w805 -> [w820]
          shift-right: [w819] -> w806
          shift-left: w805 -> [w818]
          tunnel: w804 -> [w817] mode=indexing
          n425 = Index Array(array=w817, index #1=1 ("index"), index #2=0 ("index")) -> (element #1=w814:string, element #2=w812:string)
          n426 = Search 1D Array(1D array=w820, element=w812) -> (index of element=w813:i32)  [unwired: 1 in]
          n427 = Replace Array Subset(array=w818, new element=w814, index=w813) -> (w819:string[])
        }
        n428 = Bundle By Name(cluster=w808, "Header Labels"=w806) -> (w807:T6)
        n429 = call <vilib>:"Add State(s) to Queue__jki_lib_state_machine.vi"("State(s) in (\"\")"=w811) -> ("States Out"=w810:string)  [unwired: 14 in]
      }
      frame "Reorder Data" {
        w823 = "Time\nWatts-G\nWatts-E\nkWhr-TOTAL\nRMC Raw\nRMC Corrected\nRDB F"  # Front
        w821 = "Chamber Temp\nChamber RH\nHEAT VALUE (BTU/cuFt @ STP)\nBAROMETRIC (inHG)\nGAS TEMP\nGAS PRES (inH2O)\nGAS VOLUME (cuFt)\nkWhr-G\nkWHr-E\nV-L1\nV-L2\nI-L1\nI-L2\nI-PEAK-L1\nI-PEAK-L2\nTscale\nWeight\nRaw Weight\nCorrected Weight\nWcomp\nWbouy\nAgilent Weight\ncDAQ Weight"  # Back
        # "Rename Headers: All but time, which is used in last time/rejoin procedure"
        n430 = Unbundle By Name(w829) -> ("Header Labels"=w827:string[], "Data"=w826:dbl[][])
        n431 = for {
          N: 2 -> [_]
          tunnel: w823 -> [w836]
          shift-right: [w841] -> w825
          shift-left: w827 -> [w846]
          shift-right: [w840] -> w824
          shift-left: w826 -> [w845]
          tunnel: w821 -> [w835]
          i -> [w834]
          n432 = Equal To 0?(x=w834) -> (x = 0?=w833:bool)
          n433 = Select(t=w836, s=w833, f=w835) -> (s? t:f=w837:string)
          n434 = Spreadsheet String To Array(delimiter (Tab)="\n", format string="", spreadsheet string=w837, array type (2D Dbl)=string[] []) -> (array=w844:string[])
          n435 = case shown="False" w833 {
            tunnel: w844 -> [w847 w849]
            tunnel: [w847 w848] -> w842
            frame False {
            }
            frame True {
              n436 = Reverse 1D Array(array=w849) -> (reversed array=w848:string[])
            }
          }
          n437 = for {
            shift-right: [w855] -> w841
            shift-left: w846 -> [w856]
            shift-right: [w853] -> w840
            shift-left: w845 -> [w854]
            tunnel: w842 -> [w851] mode=indexing
            tunnel: w833 -> [w850]
            n438 = Search 1D Array(1D array=w856, element=w851) -> (index of element=w852:i32)  [unwired: 1 in]
            n439 = case shown="-1" w852 {
              tunnel: w856 -> [w868 w883]
              tunnel: [w865 w883] -> w855
              tunnel: w854 -> [w864 w884]
              tunnel: [w859 w884] -> w853
              tunnel: w852 -> [w858 _]
              tunnel: w851 -> [_ w882]
              tunnel: w850 -> [w857 _]
              frame 0, Default {
                n440 = Delete From Array(array=w864, index (col)=w858) -> (deleted portion=w862:dbl[], array with subset deleted=w863:dbl[][])  [unwired: 2 in]
                n441 = Delete From Array(array=w868, length=1, index=w858) -> (deleted portion=w867:string[], array with subset deleted=w866:string[])
                n442 = Transpose 2D Array(2D array=w863) -> (transposed array=w861:dbl[][])
                n443 = case shown="True" w857 {
                  tunnel: w867 -> [w875 w876]
                  tunnel: w866 -> [w874 w877]
                  tunnel: [w873 w881] -> w865
                  tunnel: w862 -> [w872 w878]
                  tunnel: w861 -> [w871 w879]
                  tunnel: [w870 w880] -> w860
                  frame True {
                    n444 = Build Array (concatenate)(w875, w874) -> (w873:string[])
                    n445 = Build Array (concatenate)(w872, w871) -> (w870:dbl[][])
                  }
                  frame False {
                    n446 = Build Array (concatenate)(w877, w876) -> (w881:string[])
                    n447 = Build Array (concatenate)(w879, w878) -> (w880:dbl[][])
                  }
                }
                n448 = Transpose 2D Array(2D array=w860) -> (transposed array=w859:dbl[][])
              }
              frame -1 {
                n449 = case shown="\"False\", Default" w882 {
                  tunnel: w882 -> [w885 _ _]
                  frame "False", Default {
                    n450 = Concatenate Strings("Not Found " ("message"), w885) -> (w886:string)
                    n451 = disable-structure shown="Enabled" {
                      disable-tunnel: w886 -> [w888 _]
                      frame Disabled {
                        n452 = One Button Dialog(message=w888) -> ()  [unwired: 1 in, 1 out]
                      }
                      frame Enabled {
                      }
                    }
                  }
                  frame "Agilent Weight" {
                  }
                  frame "cDAQ Weight" {
                  }
                }
              }
            }
          }
        }
        n453 = Bundle By Name(cluster=w829, "Data"=w824, "Header Labels"=w825) -> (w828:T6)
        n454 = call <vilib>:"Add State(s) to Queue__jki_lib_state_machine.vi"("State(s) in (\"\")"=w832) -> ("States Out"=w831:string)  [unwired: 14 in]
      }
      frame "Make Date-Time" {
        w901 = 60.0  # sec/min
        # "Data and header go together.  Date Time String Array have\nheader attached."
        # "Rename time header, rescale time values\nto minutes, add date string to beginning of data\nand recombine data for output."
        # "CAUTION: Must be last before rejoining, since string will make data mismatch headers."
        n455 = Unbundle By Name(w912) -> ("Data"=w895:dbl[][], "Header Labels"=w909:string[])
        n456 = global read "Global Test Variables DPT.vi" "Time Header"() -> (w910:string)
        n457 = Search 1D Array(1D array=w909, element=w910) -> (index of element=w899:i32)  [unwired: 1 in]
        n458 = Replace Array Subset(array=w909, new element="TIME (min)" ("new element/subarray"), index=w899) -> (w891:string[])
        n459 = call "Array-Get 1D Column fr 2D.vi"("2D Array Data"=w895, "column index"=w899) -> ("Column Data"=w898:dbl[])  [unwired: 13 in]
        n460 = Index Array(array=w898, index=0) -> (element=w903:dbl)
        n461 = Subtract(x=w898, y=w903) -> (x-y=w902:dbl[])
        n462 = Divide(x=w902, y=w901) -> (x/y=w900:dbl[])
        n463 = Replace Array Subset(array=w895, new element=w900, index (col)=w899) -> (w889:dbl[][])  [unwired: 1 in]
        n464 = local read "Date String"() -> (w897:string)
        n465 = Build Array("DATE" ("String"), "TIME (ABS)" ("String")) -> (w908:string[])
        n466 = call "Conv Add Seconds to Date String.vi"("Seconds Array"=w898, "Init Date String"=w897) -> ("Time Array"=w896:string[], "Date Array"=w892:string[])  [unwired: 7 in, 1 out]
        n467 = Build Array(w892, w896) -> (w907:string[][])
        n468 = Transpose 2D Array(2D array=w907) -> (transposed array=w906:string[][])
        n469 = Build Array (concatenate)(w908, w906) -> (w890:string[][])
        "Date Time String Array" <- w890
        n470 = Bundle By Name(cluster=w912, "Header Labels"=w891, "Data"=w889, "Time Date String Array"=w890) -> (w911:T6)
        n471 = call <vilib>:"Add State(s) to Queue__jki_lib_state_machine.vi"("State(s) in (\"\")"=w915) -> ("States Out"=w914:string)  [unwired: 14 in]
      }
      frame "Rejoin to File Data Out" {
        w926 = i16 3  # precision
        # "Rename time header, rescale time values\nto minutes, add date string to beginning of data\nand recombine data for output."
        # "CAUTION: Must be last before rejoining, since string will make data mismatch headers."
        n472 = Unbundle By Name(w929) -> ("File Data Out"=w927:string[][], "Time Date String Array"=w920:string[][], "Data"=w921:dbl[][], "Header Labels"=w917:string[])
        n473 = Number To Fractional String(number=w921, precision (6)=w926) -> (F-format string=w919:string[][])  [unwired: 2 in]
        n474 = Build Array (concatenate)(w917, w919) -> (w918:string[][])
        n475 = Transpose 2D Array(2D array=w920) -> (transposed array=w916:string[][])
        n476 = Transpose 2D Array(2D array=w918) -> (transposed array=w924:string[][])
        n477 = Build Array (concatenate)(w916, w924) -> (w923:string[][])
        n478 = Transpose 2D Array(2D array=w923) -> (transposed array=w922:string[][])
        n479 = Build Array (concatenate)(w927, w922) -> (w925:string[][])
        n480 = Bundle By Name(cluster=w929, "File Data Out"=w925) -> (w928:T6)
        n481 = local write "File Data Out"(w925) -> ()
        n482 = call <vilib>:"Add State(s) to Queue__jki_lib_state_machine.vi"("State(s) in (\"\")"=w932) -> ("States Out"=w931:string)  [unwired: 14 in]
      }
      frame "Plot RMC" {
        # "column of term"
        # "CAUTION: Must be last before rejoining, since string will make data mismatch headers."
        n483 = Unbundle By Name(w957) -> ("Data"=w935:dbl[][], "Header Labels"=w934:string[])  [unwired: 1 out]
        n484 = Search 1D Array(1D array=w934, element="TIME (min)" ("new element/subarray")) -> (index of element=w956:i32)  [unwired: 1 in]
        n485 = Search 1D Array(1D array=w934, element="RMC Corrected" ("Front")) -> (index of element=w953:i32)  [unwired: 1 in]
        n486 = Search 1D Array(1D array=w934, element="RDB F" ("new element/subarray")) -> (index of element=w952:i32)  [unwired: 1 in]
        n487 = Search 1D Array(1D array=w934, element="RMC Raw") -> (index of element=w946:i32)  [unwired: 1 in]
        n488 = Search 1D Array(1D array=w934, element="RMC(Wf)") -> (index of element=w936:i32)  [unwired: 1 in]
        n489 = call "Array-Get 1D Column fr 2D.vi"("2D Array Data"=w935, "column index"=w956) -> ("Column Data"=w938:dbl[])  [unwired: 13 in]
        n490 = call "Array-Get 1D Column fr 2D.vi"("2D Array Data"=w935, "column index"=w946) -> ("Column Data"=w941:dbl[])  [unwired: 13 in]
        n491 = call "Array-Get 1D Column fr 2D.vi"("2D Array Data"=w935, "column index"=w953) -> ("Column Data"=w942:dbl[])  [unwired: 13 in]
        n492 = call "Array-Get 1D Column fr 2D.vi"("2D Array Data"=w935, "column index"=w936) -> ("Column Data"=w933:dbl[])  [unwired: 13 in]
        n493 = call "Array-Get 1D Column fr 2D.vi"("2D Array Data"=w935, "column index"=w952) -> ("Column Data"=w949:dbl[])  [unwired: 13 in]
        n494 = Subtract(x=w942, y=w941) -> (x-y=w940:dbl[])
        n495 = Bundle("Column Data"=w938, "Column Data"=w949) -> (→"RDB F":T3)  [unwired: 1 in]
        n496 = Bundle("Column Data"=w938, "Column Data"=w942) -> (w947:T3)  [unwired: 1 in]
        n497 = Bundle("Column Data"=w938, "Column Data"=w941) -> (w944:T3)  [unwired: 1 in]
        n498 = Bundle("Column Data"=w938, "Column Data"=w933) -> (w939:T3)  [unwired: 1 in]
        n499 = Bundle("Column Data"=w938, w940) -> (→"Compensated - raw":cluster{"Column Data":dbl[], dbl[]})  [unwired: 1 in]
        n500 = Build Array(w947, w944, w939) -> (→"RMC Compensated":T2)
        n501 = call <vilib>:"Add State(s) to Queue__jki_lib_state_machine.vi"("State(s) in (\"\")"=w960) -> ("States Out"=w959:string)  [unwired: 14 in]
      }
      frame "Plot Energy" {
        # "column of term"
        # "CAUTION: Must be last before rejoining, since string will make data mismatch headers."
        n502 = Unbundle By Name(w991) -> ("Data"=w972:dbl[][], "Header Labels"=w973:string[])  [unwired: 1 out]
        n503 = Search 1D Array(1D array=w973, element="TIME (min)" ("new element/subarray")) -> (index of element=w990:i32)  [unwired: 1 in]
        n504 = Search 1D Array(1D array=w973, element="kWhr-TOTAL" ("new element/subarray")) -> (index of element=w988:i32)  [unwired: 1 in]
        n505 = Search 1D Array(1D array=w973, element="Watts-G") -> (index of element=w977:i32)  [unwired: 1 in]
        n506 = Search 1D Array(1D array=w973, element="Watts-E") -> (index of element=w978:i32)  [unwired: 1 in]
        n507 = Search 1D Array(1D array=w973, element="kWHr-E") -> (index of element=w984:i32)  [unwired: 1 in]
        n508 = Search 1D Array(1D array=w973, element="kWhr-G" ("new element/subarray")) -> (index of element=w985:i32)  [unwired: 1 in]
        n509 = call "Array-Get 1D Column fr 2D.vi"("2D Array Data"=w972, "column index"=w990) -> ("Column Data"=w971:dbl[])  [unwired: 13 in]
        n510 = call "Array-Get 1D Column fr 2D.vi"("2D Array Data"=w972, "column index"=w988) -> ("Column Data"=w970:dbl[])  [unwired: 13 in]
        n511 = call "Array-Get 1D Column fr 2D.vi"("2D Array Data"=w972, "column index"=w977) -> ("Column Data"=w961:dbl[])  [unwired: 13 in]
        n512 = call "Array-Get 1D Column fr 2D.vi"("2D Array Data"=w972, "column index"=w984) -> ("Column Data"=w966:dbl[])  [unwired: 13 in]
        n513 = call "Array-Get 1D Column fr 2D.vi"("2D Array Data"=w972, "column index"=w978) -> ("Column Data"=w964:dbl[])  [unwired: 13 in]
        n514 = call "Array-Get 1D Column fr 2D.vi"("2D Array Data"=w972, "column index"=w985) -> ("Column Data"=w965:dbl[])  [unwired: 13 in]
        n515 = Array Max & Min(array=w970) -> (max value=→"Total kWH":dbl)  [unwired: 3 out]
        n516 = Bundle("Column Data"=w971, "Column Data"=w961) -> (→"Gas Watts":T3)  [unwired: 1 in]
        n517 = Bundle("Column Data"=w971, "Column Data"=w970) -> (→"Total kWH":T3)  [unwired: 1 in]
        n518 = Bundle("Column Data"=w971, "Column Data"=w966) -> (→"Electric kWH":T3)  [unwired: 1 in]
        n519 = Bundle("Column Data"=w971, "Column Data"=w964) -> (→"Electric Watts":T3)  [unwired: 1 in]
        n520 = Bundle("Column Data"=w971, "Column Data"=w965) -> (→"Gas kWH":T3)  [unwired: 1 in]
        n521 = call-poly <vilib>:"Mean.vi"("X"=w961) -> ("mean"=→"Ave Gas Watts":dbl)  [unwired: 1 out]
        n522 = call-poly <vilib>:"Mean.vi"("X"=w964) -> ("mean"=→"Ave Elect Watts":dbl)  [unwired: 1 out]
        n523 = Array Max & Min(array=w966) -> (max value=→"Elec kWH":dbl)  [unwired: 3 out]
        n524 = Array Max & Min(array=w965) -> (max value=→"Gas kWH 2":dbl)  [unwired: 3 out]
        n525 = call <vilib>:"Add State(s) to Queue__jki_lib_state_machine.vi"("State(s) in (\"\")"=w994) -> ("States Out"=w993:string)  [unwired: 14 in]
      }
      frame "Save Data" {
        n526 = Unbundle By Name(w998) -> ("File Data Out"=w997:string[][])
        n527 = case shown="True" "Write Eng File?" {
          tunnel: w997 -> [_ w1017]
          frame False {
          }
          frame True {
            w1024 = ".csv"  # required file extension
            n528 = local read "log file path in"() -> (w1026:path)
            n529 = Path To String(path=w1026) -> (string=w1025:string)
            n530 = Concatenate Strings("Filename Suffix", w1024) -> (w1022:string)
            n531 = Search and Replace String(input string=w1025, search string=w1024, replace string=w1022) -> (result string=w1021:string)  [unwired: 5 in, 3 out]
            n532 = String To Path(string=w1021) -> (path=w1020:path)
            n533 = call-poly <vilib>:"Write To Spreadsheet File.vi"("delimiter (\\t)"="," ("delimiter (\\t)"), "2D data"=w1017, "file path (dialog if empty)"=w1020) -> ("new file path (Not A Path if cancelled)"=→"new file path out":path)  [unwired: 5 in]
          }
        }
        n534 = case shown="True" "Write Analysis File" {
          frame False {
          }
          frame True {
            n535 = local read "FMC (lbs) Predicted"() -> (w1010:dbl)
            n536 = local read "Measured IMC"() -> (w1013:dbl)
            n537 = local read "Empty Dryer Wt"() -> (w1015:dbl)
            n538 = local read "FMC (lbs)"() -> (w1012:dbl)
            n539 = local read "FMC %"() -> (w1011:dbl)
            n540 = local read "BDW"() -> (w1014:dbl)
            n541 = local read "File Name String"() -> (w1009:string)
            n542 = Build Array(w1015, w1014, w1013, w1012, w1011, w1010) -> (w1008:dbl[])
            n543 = Array To Spreadsheet String(delimiter (Tab)=",", array=w1008, 3:"" ("format string")) -> (spreadsheet string=w1007:string)
            n544 = Build Array(w1009, w1007) -> (w1002:string[])
            n545 = call-poly <vilib>:"Write To Spreadsheet File.vi"("delimiter (\\t)"="," ("delimiter (\\t)"), "append to file? (new file:F)"=TRUE, "1D data"=w1002, "file path (dialog if empty)"="analysis file") -> ()  [unwired: 4 in, 1 out]
          }
        }
        n546 = call <vilib>:"Add State(s) to Queue__jki_lib_state_machine.vi"("State(s) in (\"\")"=w1001) -> ("States Out"=w1000:string)  [unwired: 14 in]
      }
      frame "-----Debug Data---------" {
        # "Template Separator\n(You can make a copy of, or modify, this frame)"
        n547 = call <vilib>:"Add State(s) to Queue__jki_lib_state_machine.vi"("State(s) in (\"\")"=w1030) -> ("States Out"=w1029:string)  [unwired: 14 in]
      }
      frame "Process Debug" {
        # "Parse debug log gets all data after Machine Run."
        n548 = case shown="True" "Process Debug?" {
          tunnel: w1033 -> [w1037 w1068]
          tunnel: [w1037 w1067] -> w1032
          frame False {
          }
          frame True {
            w1042 = 5  # INDEX OF ERROR MARKERS
            w1041 = 2  # COLUMNS OF ERROR MARKERS
            w1046 = 0 ("index")
            w1050 = 0  # column of count
            # "Truncate debug to length of data"
            # "Add headers"
            # "length(cols)"
            n549 = Unbundle By Name(w1068) -> ("Time Date String Array"=w1059:string[][], "Data"=w1054:dbl[][], "Header Labels"=w1071:string[])  [unwired: 1 out]
            n550 = Open/Create/Replace File(file path (use dialog)="debug log path in", access (0:read/write)=enum16{"read/write", "read-only", "write-only"}."read-only") -> (refnum out=w1077:refnum<file>, error out=w1079:errorcluster)  [unwired: 4 in, 1 out]
            n551 = Read from Text File(file (use dialog)=w1077, error in=w1079) -> (refnum out=w1075:refnum<file>, text=w1074:string, error out=w1076:errorcluster)  [unwired: 2 in, 1 out]
            n552 = Close File(refnum=w1075, error in=w1076) -> (error out=→"error out":errorcluster)  [unwired: 1 out]
            n553 = call "Parse Debug Log.vi"("text"=w1074) -> ("Headers for Data"=w1069:string[], "Array [raw rod, filt rod, outlet t, inlet t, coil, curve or hr]"=w1073:i32[][], "Time Array"=w1062:string[])  [unwired: 8 in]
            "Headers for Debug Data" <- w1069
            n554 = Build Array (concatenate)("Debug Time" ("Current State"), w1062) -> (w1060:string[])
            "Debug Time Array" <- w1060
            n555 = To Double Precision Float(number=w1073) -> (double precision float=w1043:dbl[][])
            "Debug Data" <- w1043
            n556 = Array Subset(array=w1043, index (col)=w1042, length (col)=w1041) -> (w1040:dbl[][])  [unwired: 2 in]
            n557 = call "Array-Add 1D Str Column to 2D.vi"("Column to Add"=w1060, "Original Array"=w1059) -> ("Result Array"=w1052:string[][])  [unwired: 9 in]
            n558 = Greater Than 0?(x=w1040) -> (x > 0?=w1039:bool[][])
            n559 = Or Array Elements(Boolean array=w1039) -> (logical OR=→"Error Indicated in Last 2cols\nof Debug Log":bool)
            n560 = Array Size(array=w1054) -> (size(s)=w1058:i32[])
            n561 = Delete From Array(array=w1043, index (col)=w1050) -> (deleted portion=w1048:dbl[])  [unwired: 2 in, 1 out]
            n562 = Index Array(array=w1058, index=0) -> (element=w1056:i32)
            n563 = Array Subset(array=w1043, index (row)=0 ("index"), length (row)=w1056) -> (w1055:dbl[][])  [unwired: 2 in]
            n564 = Build Array (concatenate)(w1071, w1069) -> (w1070:string[])
            n565 = local write "Date Time String Array"(w1052) -> ()
            n566 = Delete From Array(array=w1048, length=1, index=w1046) -> (array with subset deleted=w1045:dbl[])  [unwired: 1 out]
            n567 = Index Array(array=w1048, index=w1046) -> (element=w1049:dbl)
            n568 = Transpose 2D Array(2D array=w1054) -> (transposed array=w1053:dbl[][])
            n569 = Transpose 2D Array(2D array=w1055) -> (transposed array=w1064:dbl[][])
            n570 = Build Array (concatenate)(w1053, w1064) -> (w1063:dbl[][])
            n571 = for {
              shift-right: [w1082] -> _
              shift-left: w1049 -> [w1083]
              tunnel: w1045 -> [w1082] mode=indexing
              tunnel: [w1084] -> w1044 mode=indexing
              n572 = Subtract(x=w1082, y=w1083) -> (x-y=w1084:dbl)
            }
            "Com Count (x(k+1)-x(k))" <- w1044
            n573 = Transpose 2D Array(2D array=w1063) -> (transposed array=w1072:dbl[][])
            n574 = Bundle By Name(cluster=w1068, "Time Date String Array"=w1052, "Header Labels"=w1070, "Data"=w1072) -> (w1067:T6)
            n575 = flat-sequence {
              tunnel: w1044 -> [_]
              frame #0 {
                n576 = property on="Com Count (x(k+1)-x(k))" class="WFGraph (strict)"("YScale.Maximum"=5.0 ("Y Scale.Range:Maximum"), "YScale.Minimum"=-1.0 ("Y Scale.Range:Minimum")) -> ()  [unwired: 2 in, 2 out]
              }
            }
          }
        }
        n577 = call <vilib>:"Add State(s) to Queue__jki_lib_state_machine.vi"("State(s) in (\"\")"=w1036) -> ("States Out"=w1035:string)  [unwired: 14 in]
      }
      frame "--------Functions------------" {
        # "Template Separator\n(You can make a copy of, or modify, this frame)"
        n578 = call <vilib>:"Add State(s) to Queue__jki_lib_state_machine.vi"("State(s) in (\"\")"=w1088) -> ("States Out"=w1087:string)  [unwired: 14 in]
      }
      frame "Replace Data Out Term" {
        # "Replace Data Out Term >> &term, value"
        n579 = Unbundle By Name(w1099) -> ("File Data Out"=w1096:string[][])
        n580 = Match Pattern(string=w1092, regular expression=",") -> (before substring=w1090:string, after substring=w1089:string)  [unwired: 1 in, 2 out]
        n581 = Array To Spreadsheet String(array=w1096, 3:"" ("format string")) -> (spreadsheet string=w1095:string)  [unwired: 1 in]
        n582 = Search and Replace String(input string=w1095, search string=w1090, replace string=w1089) -> (result string=w1094:string)  [unwired: 5 in, 3 out]
        n583 = flat-sequence {
          tunnel: w1094 -> [w1104]
          tunnel: [w1103] -> w1093
          frame #0 {
            w1105 = "" ("format string")
            n584 = Spreadsheet String To Array(format string=w1105, spreadsheet string=w1104, array type (2D Dbl)=w1105) -> (array=w1103:string[][])  [unwired: 1 in]
            n585 = local write "File Data Out"(w1103) -> ()
          }
        }
        n586 = Bundle By Name(cluster=w1099, "File Data Out"=w1093) -> (w1098:T6)
        n587 = call <vilib>:"Add State(s) to Queue__jki_lib_state_machine.vi"("State(s) in (\"\")"=w1102) -> ("States Out"=w1101:string)  [unwired: 14 in]
      }
    }
    n588 = Equal To 0?(x=w10) -> (x = 0?=w9:bool)
    n589 = disable-structure shown="Enabled" {
      disable-tunnel: w11 -> [w24 _]
      disable-tunnel: w9 -> [w23 _]
      frame Disabled {
        n590 = call "Build String Array.vi"("Initialize"=w23, "string"=w24) -> ("Array"=→"Array":string[])  [unwired: 9 in]
      }
      frame Enabled {
        # "for Debug"
      }
    }
    n591 = Tick Count (ms)() -> (millisecond timer value=w8:u32)
  }
  "Timeing" <- w3
  n592 = Unbundle By Name(w5) -> ("File Data Out"=→"File Data Out":string[][], "error in"=→"error out":errorcluster)
